vi "2.0.0_BEMF_Calibration.vi"(6 ".bat":T1={"getVersion"="Getting Software Version.bat", "Start Test mode"="Start Test Mode.bat", "Start camera test mode"="Start camera test mode.bat", "get one RAW Image"="Get one image.bat", "Stop camera test mode"="Stop camera test mode.bat", "Stop Test Mode"="Stop Test Mode.bat", "Get image reflection"="Get image reflection.bat", "Get image uniformity andFlash LED brightness"="Get image uniformity andFlash LED brightness.bat", "Disable flash LED"="Disable flash LED.bat", "Enable flash LED"="Enable flash LED.bat", "Software Reset"="Software Reset.bat", "Tune Flash LED brightness"="Tune Flash LED brightness.bat", "Start Camera calibration"="Start Camera calibration.bat", "Verify OBC Setting"="Verify OBC Setting.bat"}, 7 "Data in":T3, 8 "error in (no error)":errorcluster, 9 "AllControls In":T2, 11 "Message Queue out":T4) -> (0 "error out":errorcluster, 1 "Flow":string, 3 "Message Queue Out":T4, 5 "Data out":T3)   [LabVIEW 2017]
uses:
  Depends/AMC/subVIs/TypeDefs/amc_Message Queue.ctl
  Depends/AMC/subVIs/TypeDefs/amc_Message.ctl
  Depends/Tools/Keyed Array/Tools_KeyedArray KeyedArray.ctl
  Ctrls/CSV_Data.ctl
  Ctrls/AllControls.ctl
  Ctrls/NFC.bat
panel:
  out "GetImage?":bool
  out "retry_flag":bool
  in  "Num":i32
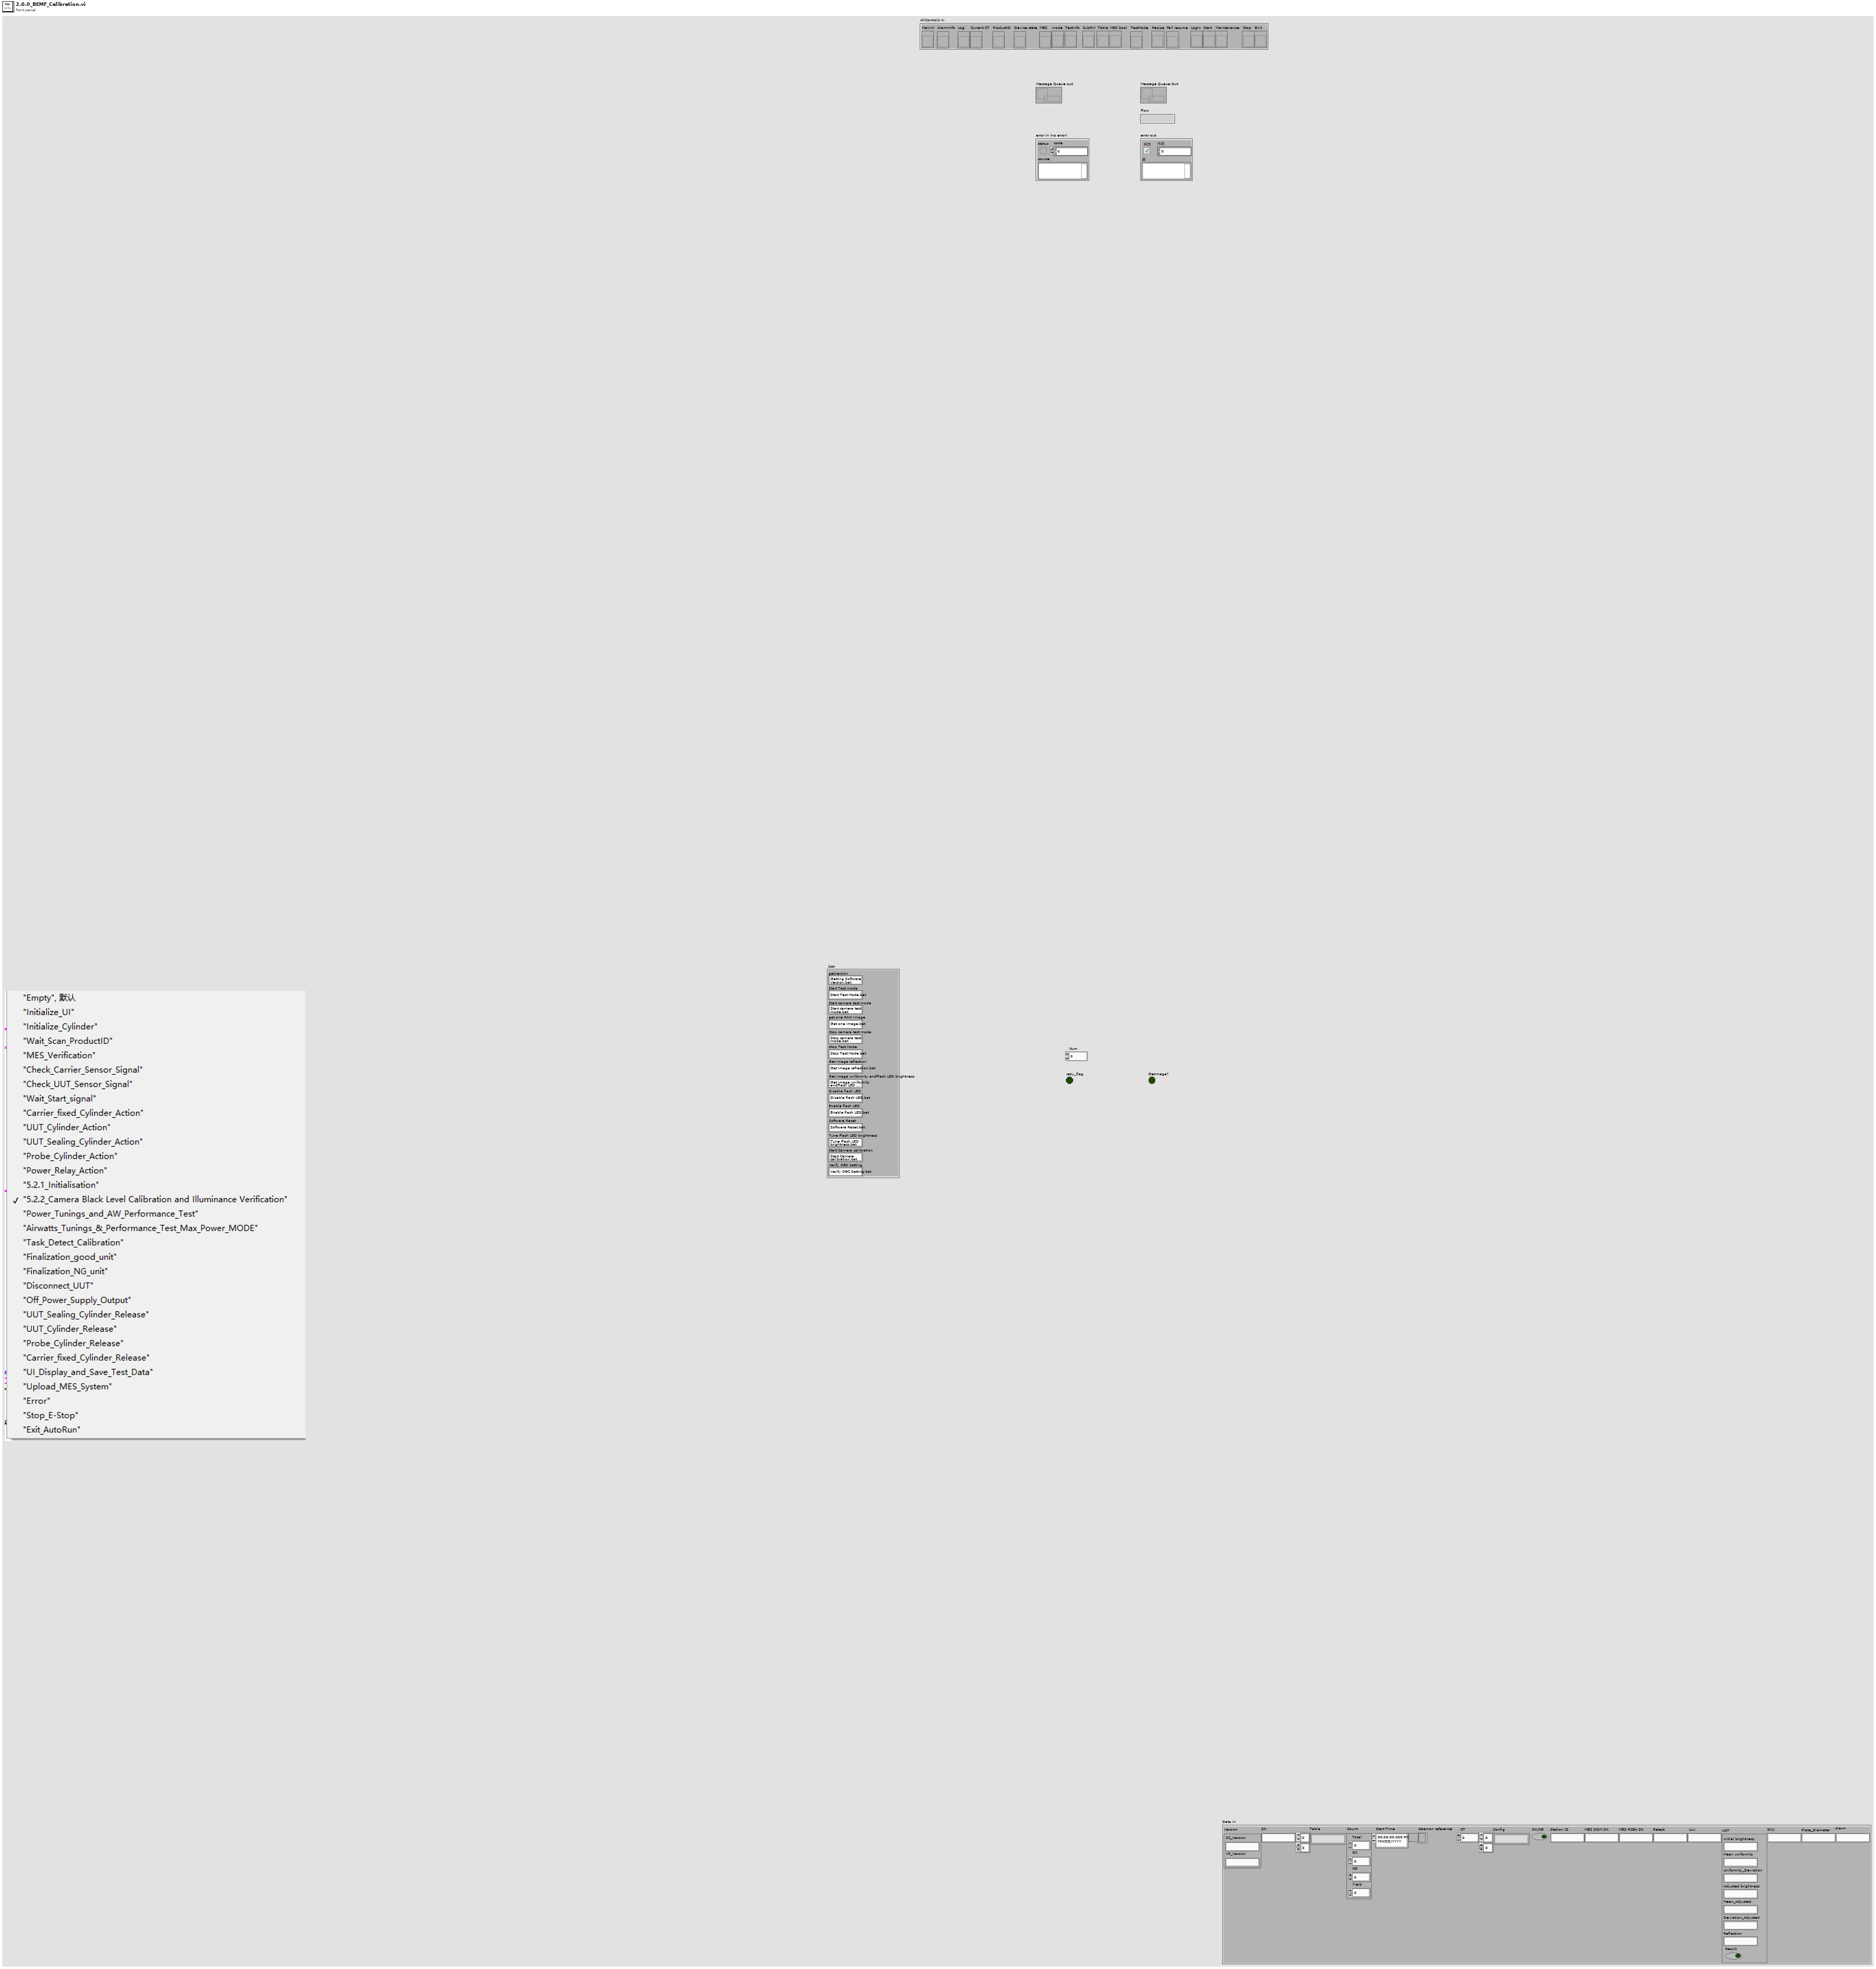
[diagram p1: front panel]
types:
  T1 = typedef "NFC.bat" = cluster{"getVersion":string, "Start Test mode":string, "Start camera test mode":string, "get one RAW Image":string, "Stop camera test mode":string, "Stop Test Mode":string, "Get image reflection":string, "Get image uniformity andFlash LED brightness":string, "Disable flash LED":string, "Enable flash LED":string, "Software Reset":string, "Tune Flash LED brightness":string, "Start Camera calibration":string, "Verify OBC Setting":string}
  T2 = typedef "AllControls.ctl" = cluster{"MainVI":refnum<vi>, "AlarmInfo":refnum<vi>, "Log":refnum<vi>, "Current CT":refnum<vi>, "ProductID":refnum<vi>, "Device state":refnum<vi>, "MES":refnum<vi>, "mode":refnum<vi>, "TestInfo":refnum<vi>, "SubPnl":refnum<vi>, "Table":refnum<vi>, "MES bool":refnum<vi>, "TestMode":refnum<vi>, "Recipe":refnum<vi>, "Fail resume":refnum<vi>, "LogIn":refnum<vi>, "Start":refnum<vi>, "Maintenance":refnum<vi>, "Stop":refnum<vi>, "Exit":refnum<vi>}
  T3 = typedef "CSV_Data.ctl" = cluster{"Version":cluster{"SC_Version":string, "VP_Version":string}, "SN":string, "Table":string[][], "Count":cluster{"Total":i32, "OK":i32, "NG":i32, "Yield":dbl}, "Start Time":timestamp, "daemon reference":refnum<k5>, "CT":dbl, "Config":string[][], "OK/NG":bool, "Station ID":string, "MES DDM SN":string, "MES PCBA SN":string, "Retest":string, "Lux":string, "VOT":cluster{"Initial brightness":string, "Mean uniformity":string, "Uniformity_Deviation":string, "Adjusted brightness":string, "Mean_Adjusted":string, "Deviation_Adjusted":string, "Reflection":string, "Result":bool}, "SKU":string, "Plate_Diameter":string, "Alarm":string}
  T4 = typedef "amc_Message Queue.ctl" = refnum<queue>
  T5 = typedef "HD Config.ctl" = cluster{" PC":cluster{"PC Address":u8[], "PC Port":i32}, "FCO":cluster{"COM":refnum<visa-resource-name>, "Baudrate":u32}, "DC Power ":cluster{"COM":refnum<visa-resource-name>, "Baudrate":u32}, "PW3336":cluster{"COM":refnum<visa-resource-name>, "Baudrate":u32}, "Lefoo":cluster{"COM":refnum<visa-resource-name>, "Baudrate":u32}, "Tempt&Hum":cluster{"COM":refnum<visa-resource-name>, "Baudrate":u32}, "DIPC":cluster{"COM":refnum<visa-resource-name>}, "Daemon":cluster{"IP Address":string, "Port":u16, "Retry":u16}, "NFC_Cmd":cluster{"COM":refnum<visa-resource-name>, "Baudrate":u32}, "Fail_resume_mode":bool, "GRR":bool, "NFC _Serial":cluster{"COM":refnum<visa-resource-name>, "Baudrate":u32}}
  T6 = typedef "TesterInfo.ctl" = cluster{"Station Name":string, "Station Code":string, "ES NO.":string, "Tester ID":string, "PassMark Revision":string, "Rig ID":string, "682_Tool_Repeat":string, "Project Name":string, "FFTesterPath":path, "Enable_User":bool, "Mode":enum16{"682"}, "Fail_resume_mode":bool}
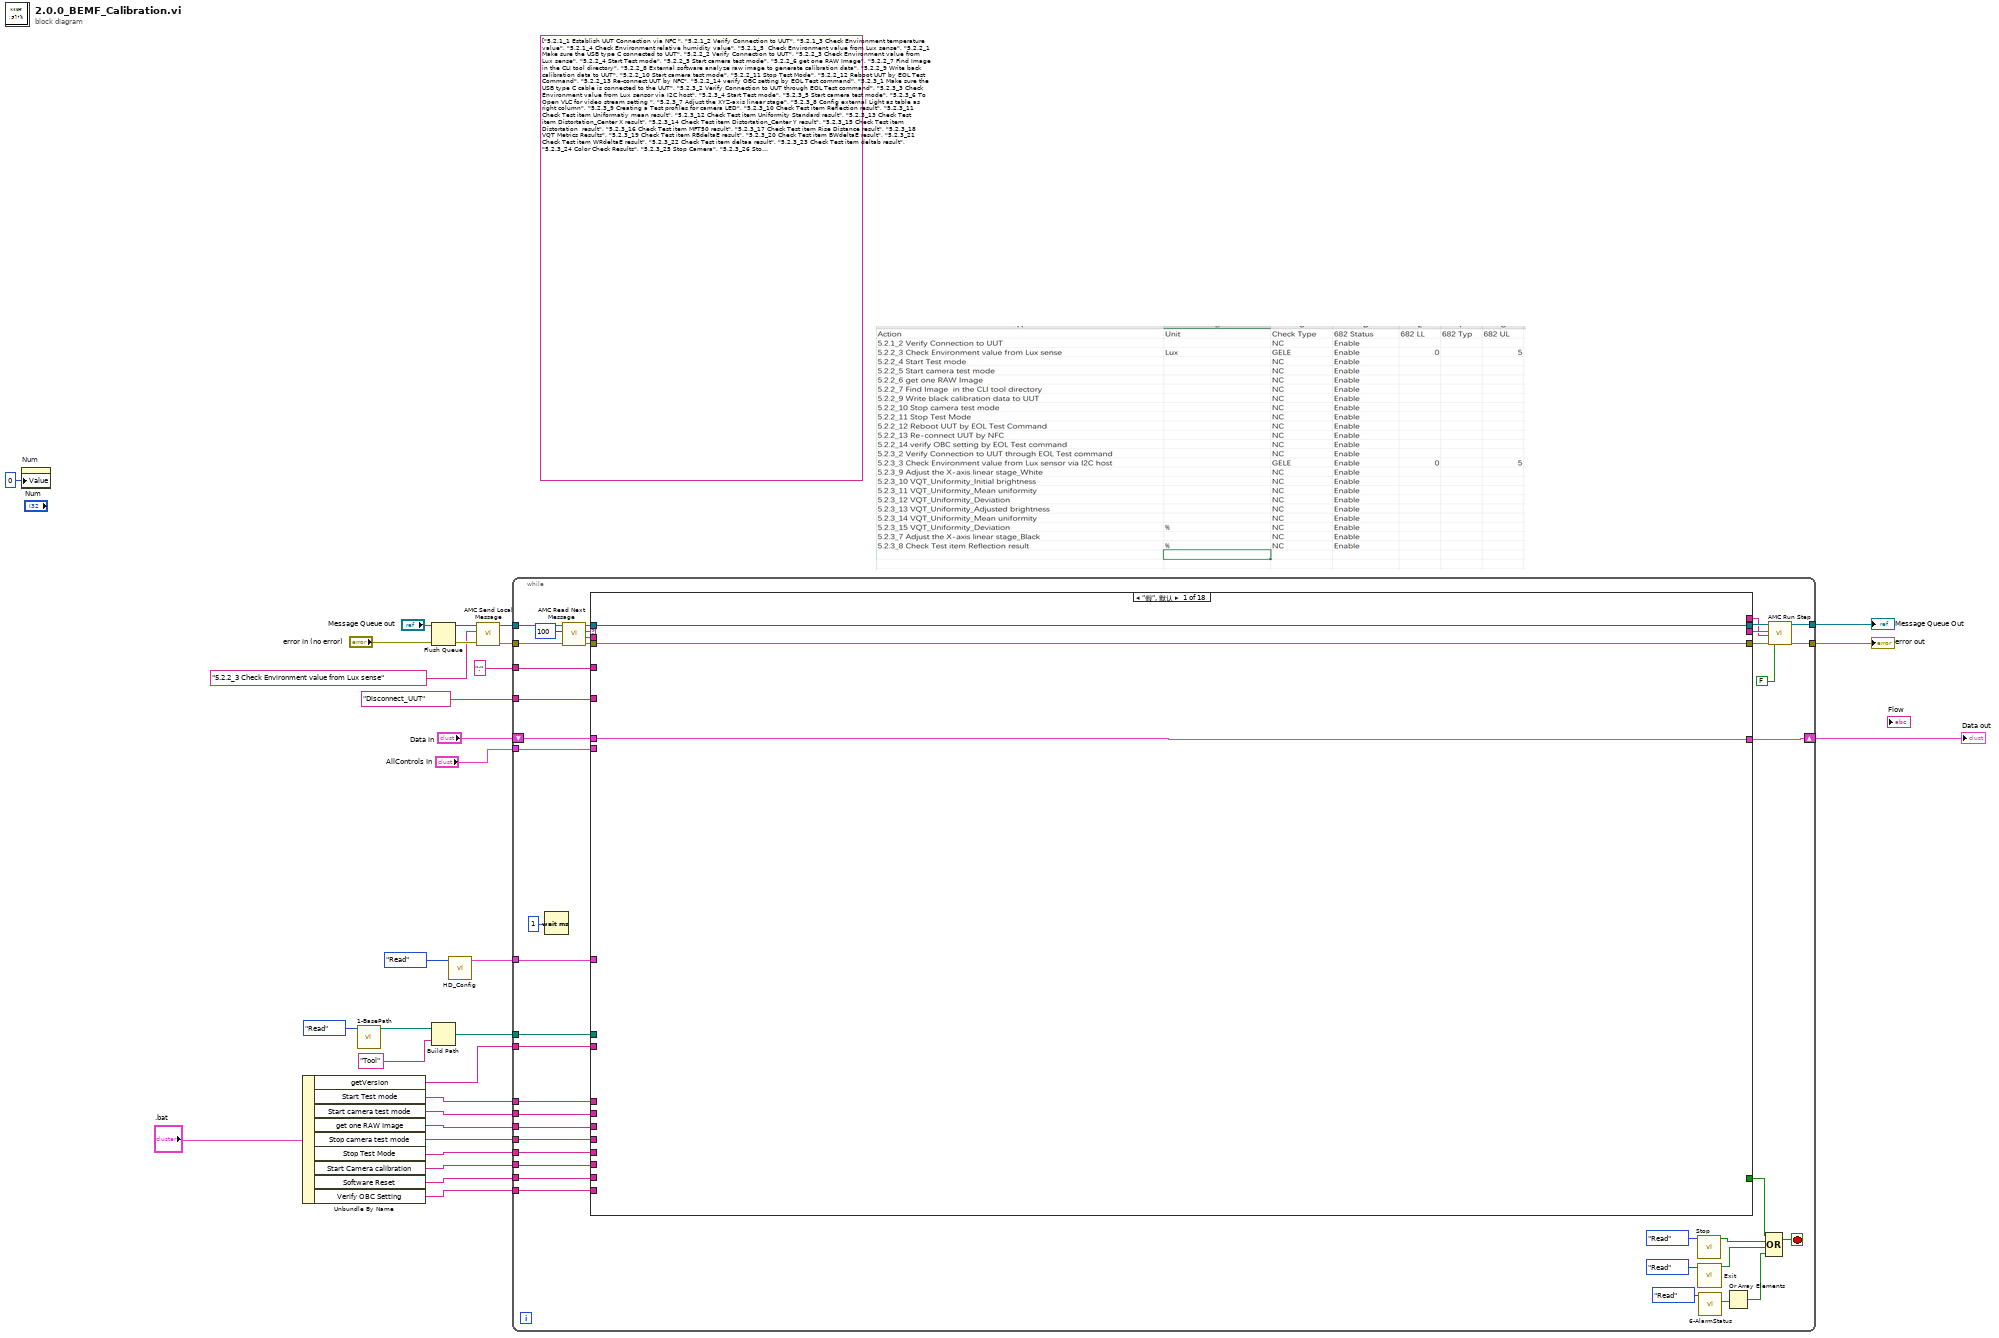
[diagram p0: block diagram]
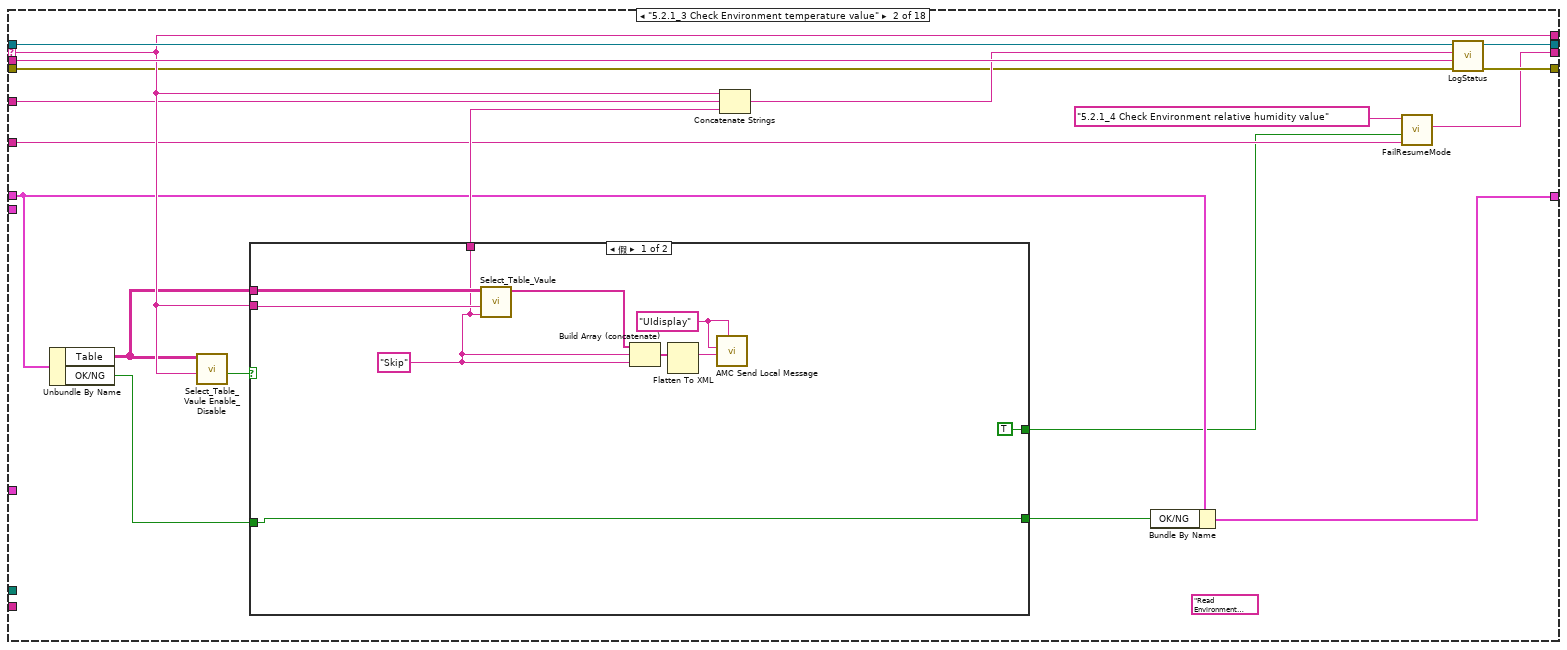
[diagram p2: hidden frame]
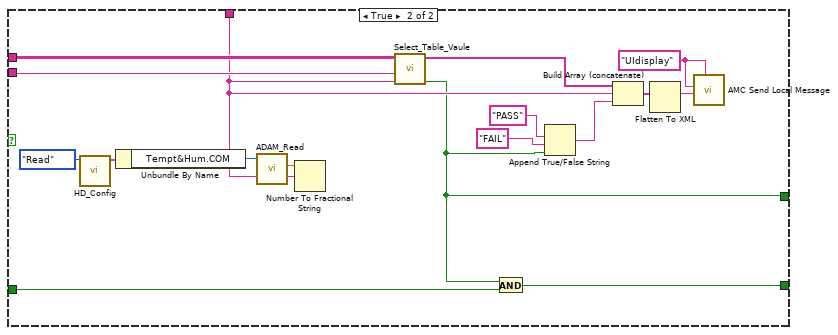
[diagram p3: hidden frame]
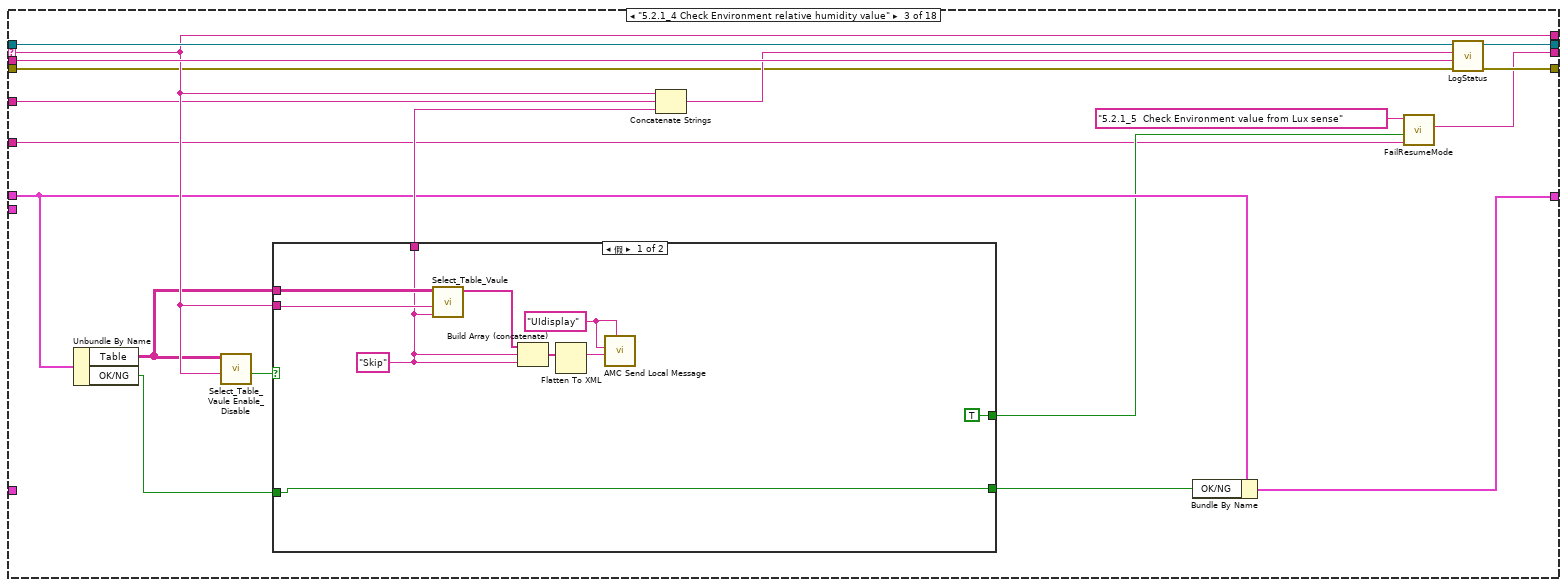
[diagram p4: hidden frame]
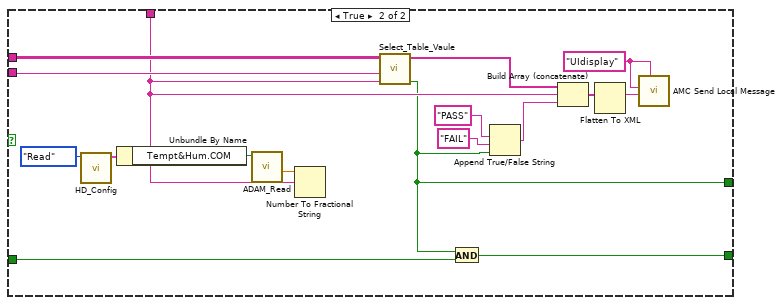
[diagram p5: hidden frame]
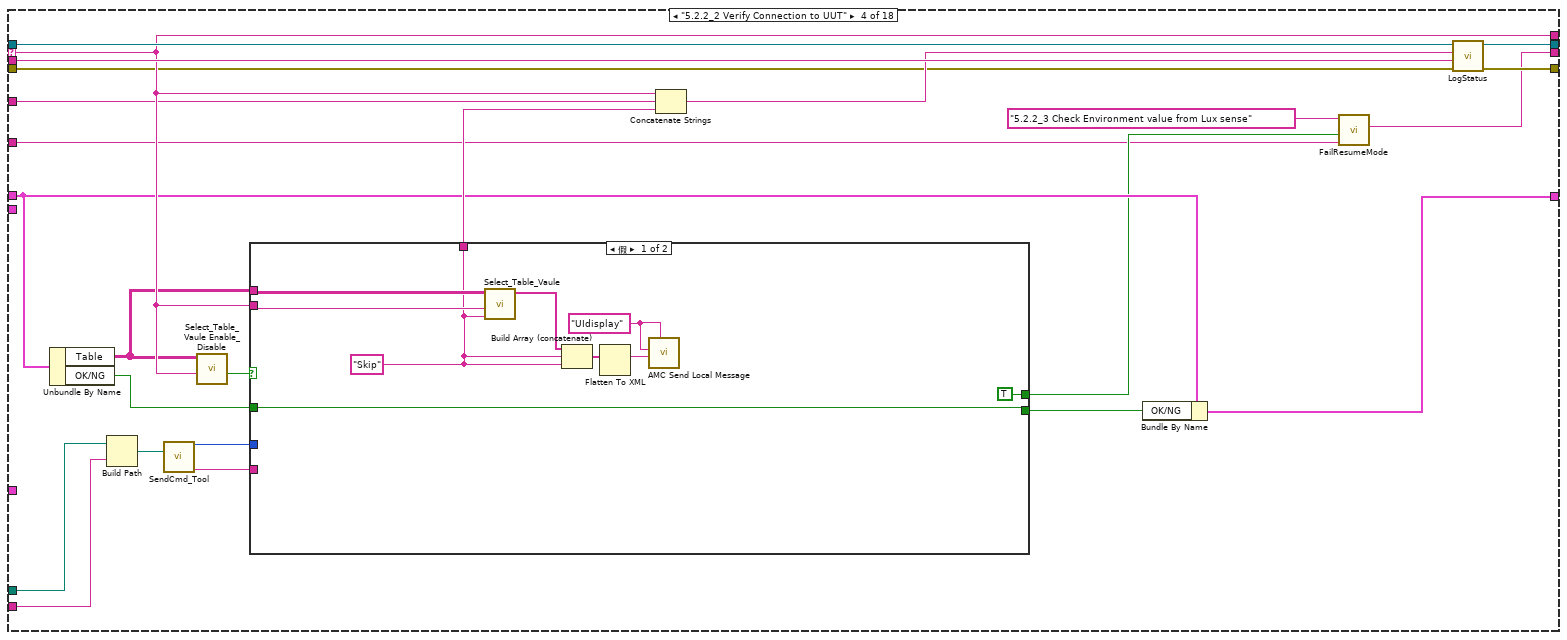
[diagram p6: hidden frame]
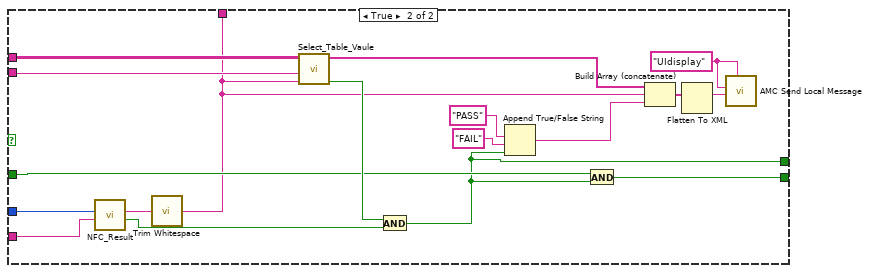
[diagram p7: hidden frame]
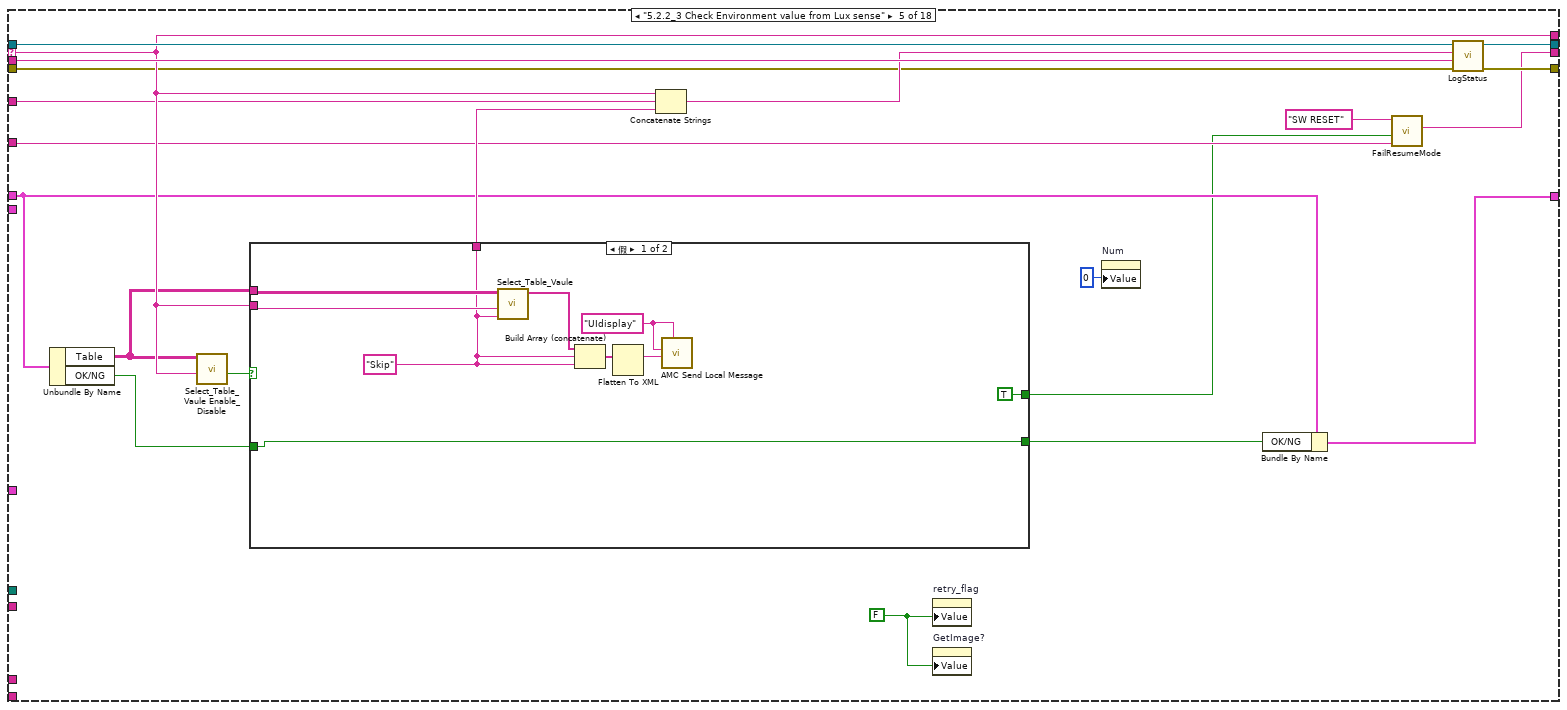
[diagram p8: hidden frame]
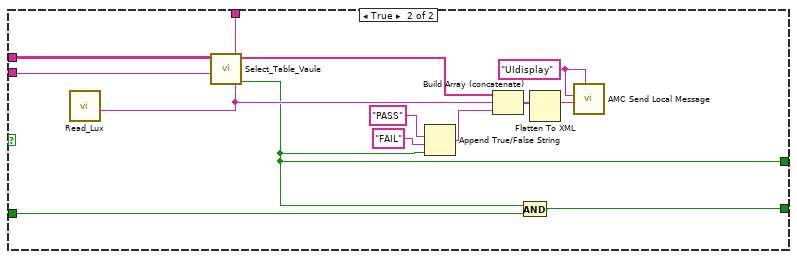
[diagram p9: hidden frame]
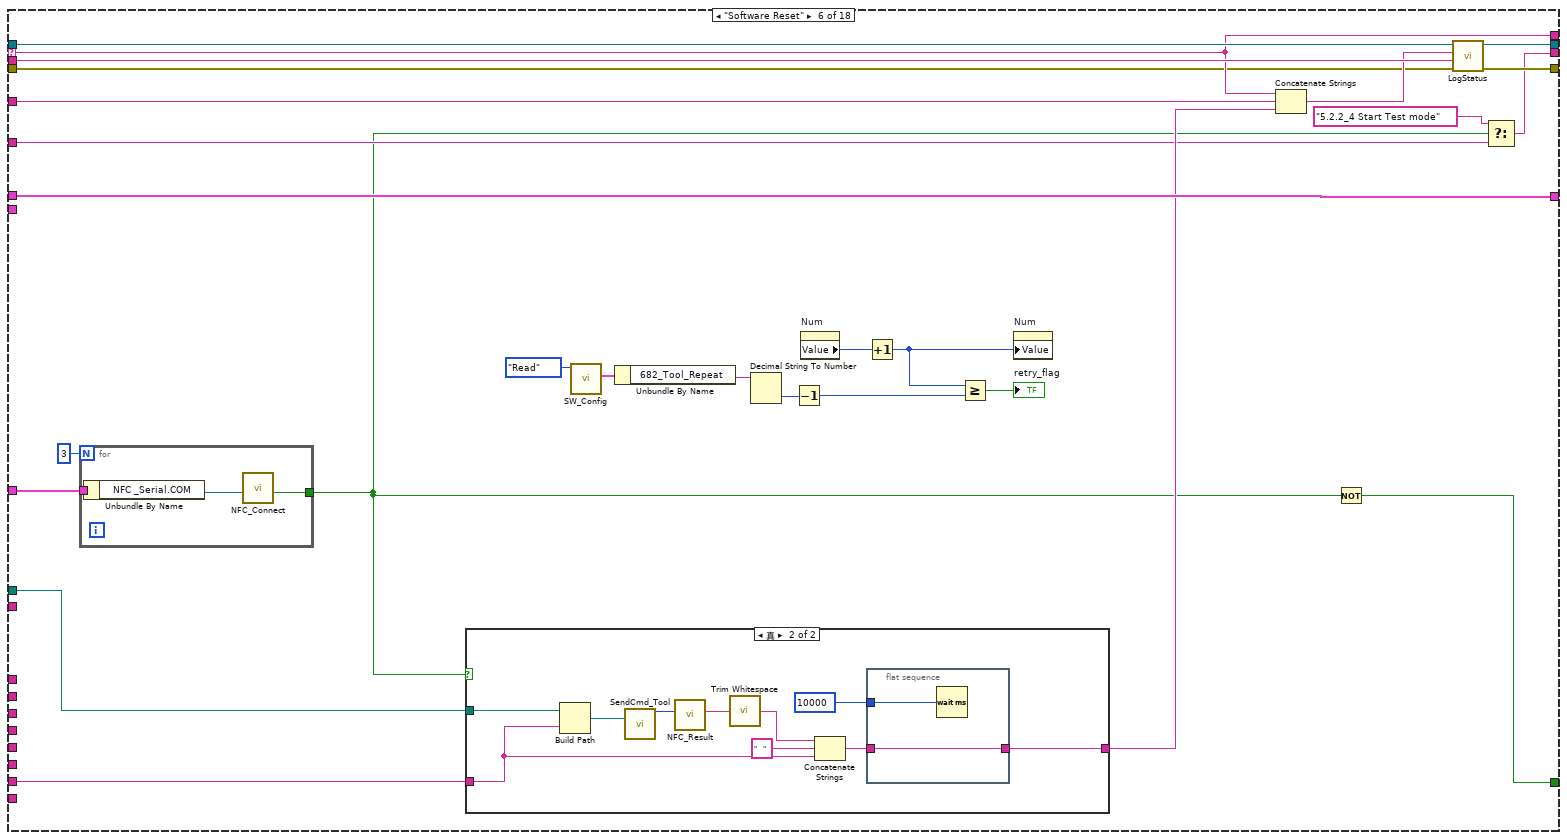
[diagram p10: hidden frame]
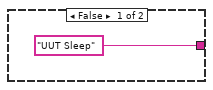
[diagram p11: hidden frame]
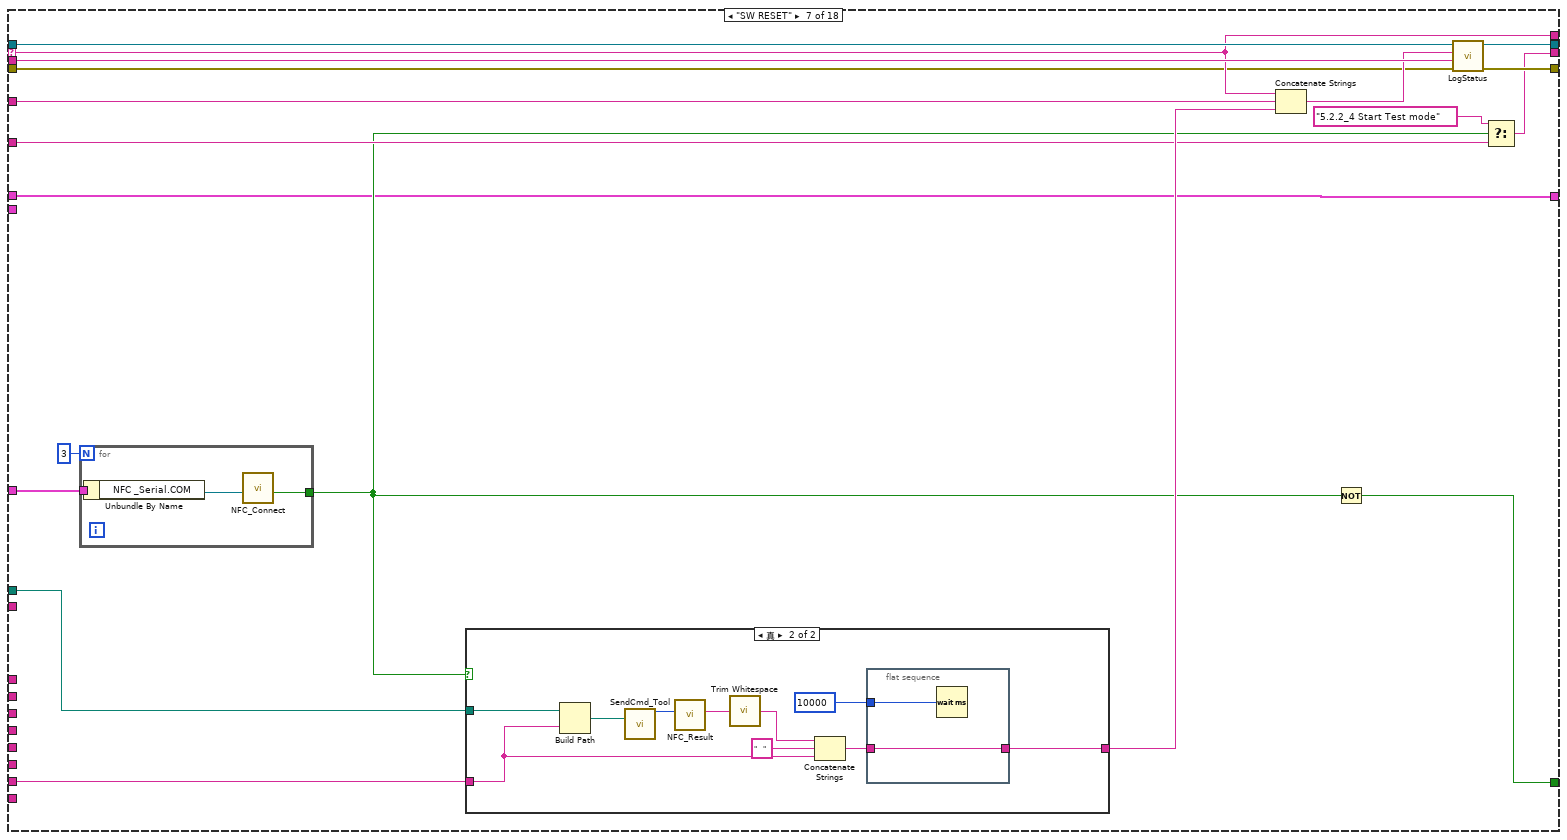
[diagram p12: hidden frame]
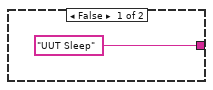
[diagram p13: hidden frame]
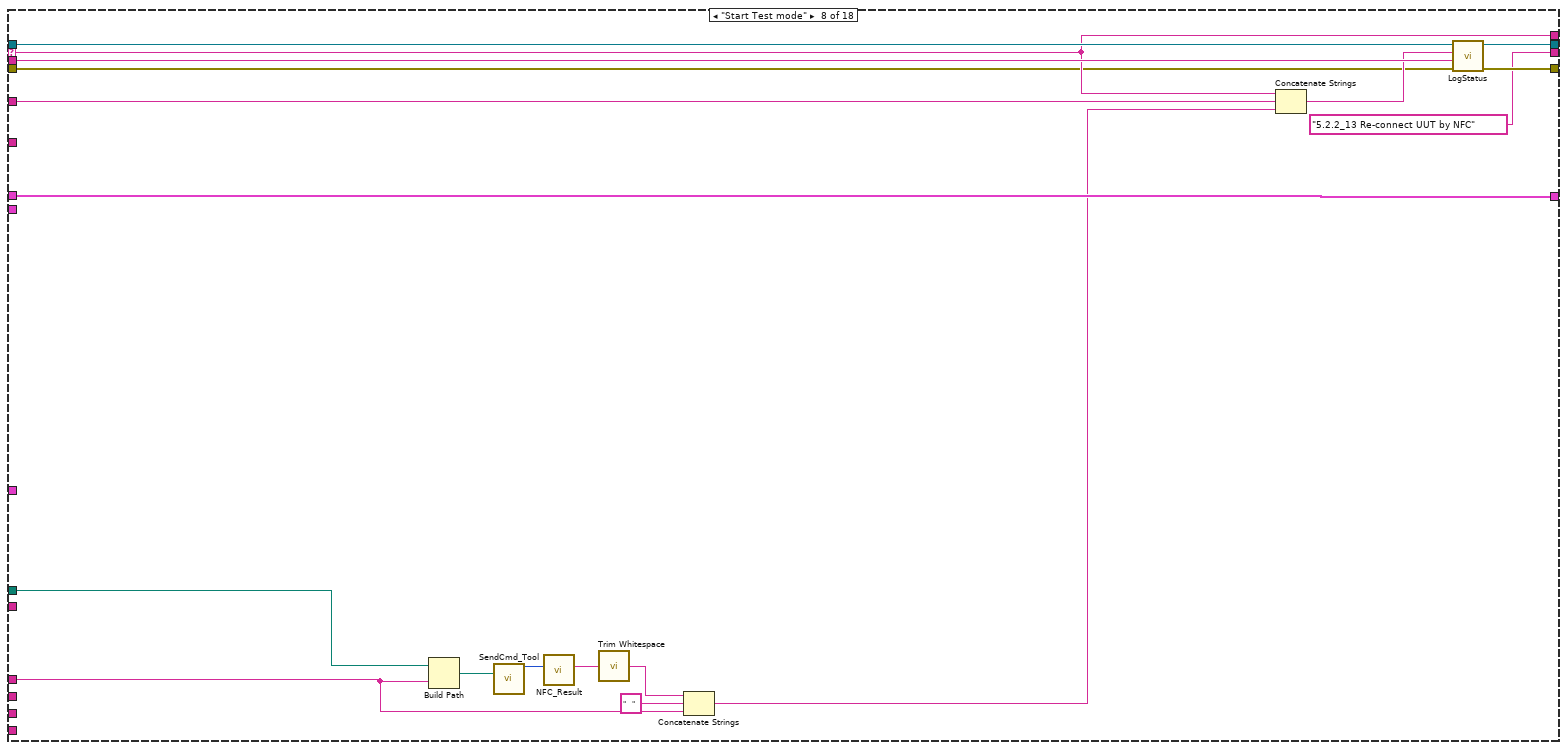
[diagram p14: hidden frame]
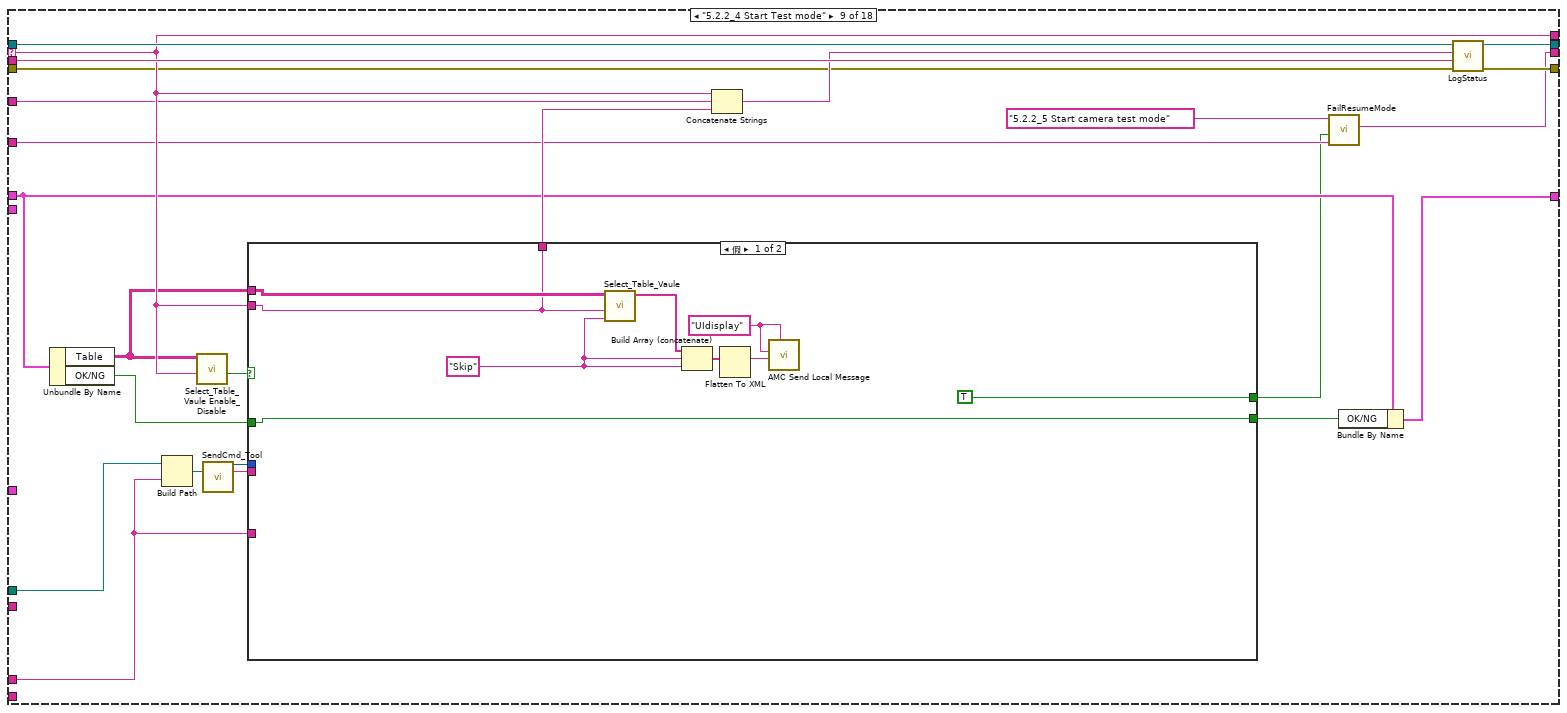
[diagram p15: hidden frame]
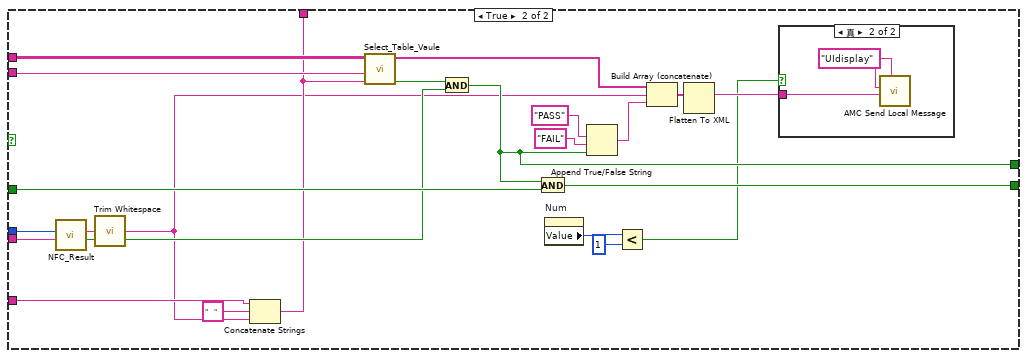
[diagram p16: hidden frame]
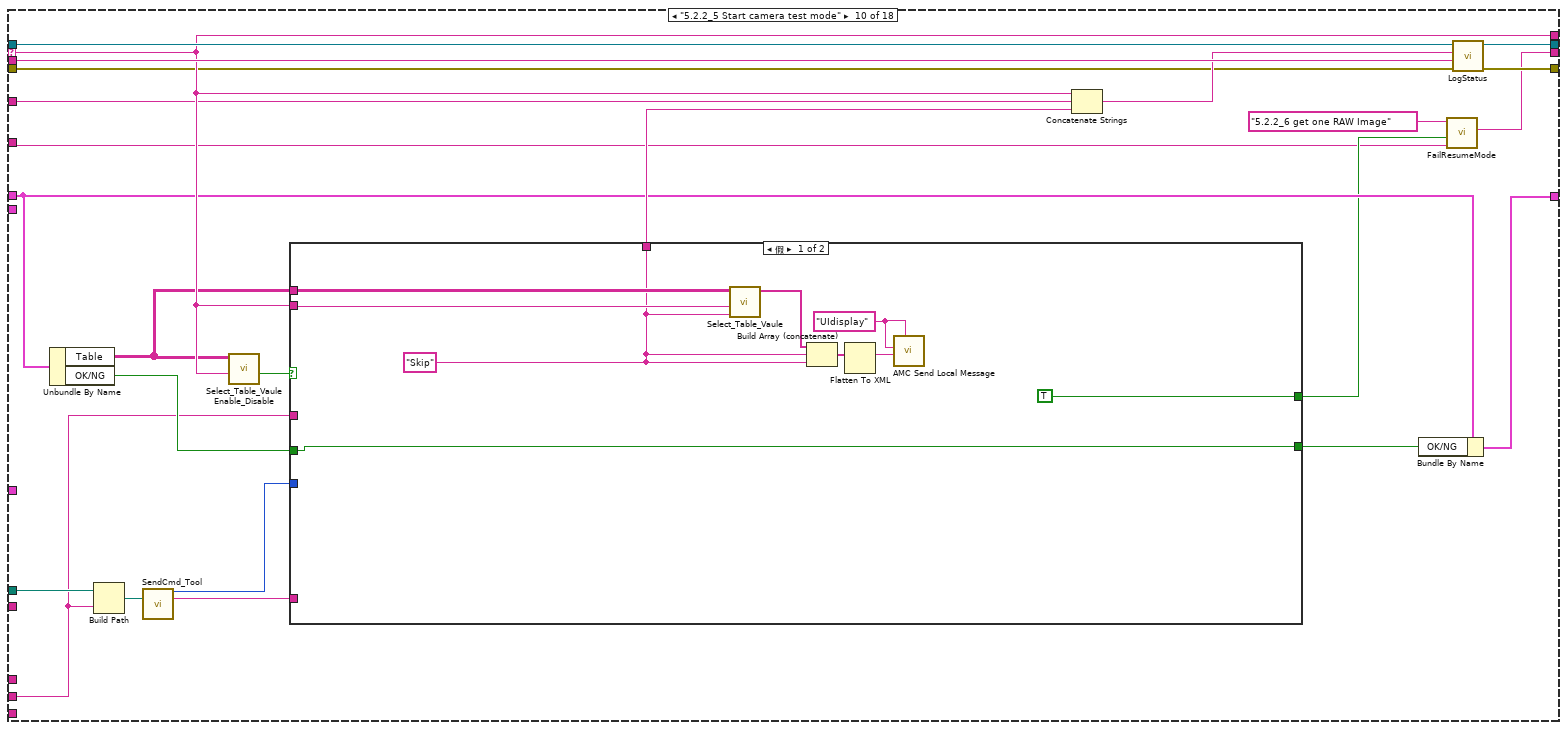
[diagram p18: hidden frame]
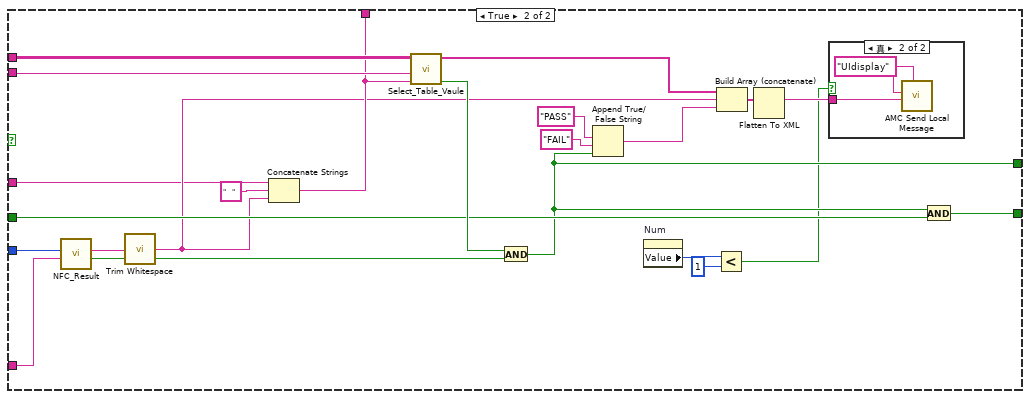
[diagram p19: hidden frame]
diagram:
  (unwired) string[] ["5.2.1_1 Establish UUT Connection via NFC ", "5.2.1_2 Verify Connection to UUT", "5.2.1_3 Check Environment temperature value", "5.2.1_4 Check Environment relative humidity value", "5.2.1_5  Check Environment value from Lux sense", "5.2.2_1 Make sure the USB type C connected to UUT", "5.2.2_2 Verify Connection to UUT", "5.2.2_3 Check Environment value from Lux sense", "5.2.2_4 Start Test mode", "5.2.2_5 Start camera test mode", "5.2.2_6 get one RAW Image", "5.2.2_7 Find Image  in the CLI tool directory", "5.2.2_8 External software analyze raw image to generate calibration data", "5.2.2_9 Write back calibration data to UUT", "5.2.2_10 Start camera test mode", "5.2.2_11 Stop Test Mode", "5.2.2_12 Reboot UUT by EOL Test Command", "5.2.2_13 Re-connect UUT by NFC", "5.2.2_14 verify OBC setting by EOL Test command", "5.2.3_1 Make sure the USB type C cable is connected to the UUT", "5.2.3_2 Verify Connection to UUT through EOL Test command", "5.2.3_3 Check Environment value from Lux sensor via I2C host", "5.2.3_4 Start Test mode", "5.2.3_5 Start camera test mode", "5.2.3_6 To Open VLC for video stream setting ", "5.2.3_7 Adjust the XYZ-axis linear stage", "5.2.3_8 Config external Light as table as right column", "5.2.3_9 Creating a Test profiles for camera LED", "5.2.3_10 Check Test item Reflection result", "5.2.3_11 Check Test item Uniformatiy mean result", "5.2.3_12 Check Test item Uniformity Standard result", "5.2.3_13 Check Test item Distortation_Center X result", "5.2.3_14 Check Test item Distortation_Center Y result", "5.2.3_15 Check Test item Distortation  result", "5.2.3_16 Check Test item MFT50 result", "5.2.3_17 Check Test item Rise Distance result", "5.2.3_18 VQT Metrics Results", "5.2.3_19 Check Test item RBdeltaE result", "5.2.3_20 Check Test item BWdeltaE result", "5.2.3_21 Check Test item WRdeltaE result", "5.2.3_22 Check Test item deltaa result", "5.2.3_23 Check Test item deltab result", "5.2.3_24 Color Check Results", "5.2.3_25 Stop Camera", "5.2.3_26 Stop Test mode", "5.2.3_27 Shutdown UUT"] ("subarray")
  n1 = property on="Num" class="DigNum (严格)"("Value"=0 ("Num")) -> ()  [unwired: 2 in, 2 out]
  n2 = Unbundle By Name(".bat") -> ("getVersion"=w14:string, "Start Test mode"=w13:string, "Start camera test mode"=w12:string, "get one RAW Image"=w11:string, "Stop camera test mode"=w10:string, "Stop Test Mode"=w9:string, "Start Camera calibration"=w6:string, "Software Reset"=w4:string, "Verify OBC Setting"=w3:string)
  n3 = call "1-BasePath.vi"("Step"=enum16{"Initial", "Write", "Read"}."Read") -> ("Path Out"=w16:path)  [unwired: 9 in, 1 out]
  n4 = Flush Queue(queue="Message Queue out") -> (queue out=w24:T4)  [unwired: 1 in, 2 out]
  n5 = Build Path(base path=w16, name or relative path="Tool") -> (appended path=w15:path)
  n6 = call "HD_Config.vi"("Step"=enum16{"Initial", "Write", "Read"}."Read") -> ("HD Config out"=w25:T5)  [unwired: 9 in, 1 out]
  n7 = call "AMC Send Local Message.vi"("error in (no error)"="error in (no error)", "Message Name"="5.2.2_3 Check Environment value from Lux sense", "Message Queue in"=w24) -> ("error out"=w28:errorcluster, "Message Queue out"=w29:T4)  [unwired: 7 in]
  n8 = while {
    tunnel: w29 -> [w70]
    tunnel: [w66] -> w23
    tunnel: w28 -> [w64]
    tunnel: [w61] -> w22
    tunnel: w25 -> [w58]
    shift-right: [w47] -> w20
    shift-left: "Data in" -> [w48]
    tunnel: "AllControls In" -> [w46]
    tunnel: w15 -> [w42]
    tunnel: w14 -> [w41]
    tunnel: w13 -> [w40]
    tunnel: w12 -> [w39]
    tunnel: w11 -> [w38]
    tunnel: w10 -> [w37]
    tunnel: w9 -> [w36]
    tunnel: ":" -> [w35]
    tunnel: "Disconnect_UUT" -> [w34]
    tunnel: w6 -> [w33]
    tunnel: w4 -> [w32]
    tunnel: w3 -> [w31]
    stop <- w49 stop-if-true
    n9 = Wait (ms)(milliseconds to wait=u32 1 ("等待时间（毫秒）")) -> ()  [unwired: 1 out]
    n10 = call "AMC Read Next Message.vi"("error in (no error)"=w64, "timeout (1ms)"=100, "Message Queue in"=w70) -> ("error out"=w63:errorcluster, "Message Value"=w56:string, "Message Name"=w68:string, "Message Queue out"=w69:T4)  [unwired: 1 in, 4 out]
    n11 = case shown="\"假\", 默认" w68 {
      selector: w68 -> [_ w85 w129 w178 w225 w275 w309 w342 w363 w420 w483 w537 w584 w638 w688 w738 w794 w846]
      tunnel: w69 -> [w73 w91 w135 w184 w231 w279 w313 w346 w369 w426 w489 w543 w590 w644 w694 w742 w799 w851]
      tunnel: [w73 w91 w135 w184 w231 w279 w313 w346 w369 w426 w489 w543 w590 w644 w694 w742 w799 w851] -> w67
      tunnel: w63 -> [w72 w79 w123 w167 w219 w274 w308 w341 w353 w410 w476 w535 w582 w627 w677 w736 w792 w843]
      tunnel: [w72 w90 w134 w183 w230 w278 w312 w345 w368 w425 w488 w542 w589 w643 w693 w741 w798 w850] -> w62
      tunnel: [_ _ _ _ _ w260 w299 _ _ _ _ _ _ _ _ _ _ TRUE] -> w50
      tunnel: w56 -> [_ w89 w133 w182 w229 w277 w311 w344 w367 w424 w487 w541 w588 w642 w692 w740 w797 w849]
      tunnel: [_ w85 w129 w178 w225 w275 w309 w342 w363 w420 w483 w537 w584 w638 w688 w738 w794 w846] -> w55
      tunnel: w58 -> [_ _ _ _ _ w264 w296 _ _ _ _ _ _ _ _ w733 w788 _]
      tunnel: [_ w75 w118 w162 w216 w262 w301 "5.2.2_13 Re-connect UUT by NFC" w349 w405 w473 w526 w568 w622 w672 w723 w781 w840] -> w57
      tunnel: w48 -> [w71 w83 w126 w170 w223 w271 w297 w338 w356 w415 w478 w532 w575 w630 w680 w728 w787 w836]
      tunnel: [w71 w80 w124 w169 w220 w271 w297 w338 w355 w414 w477 w530 w574 w629 w679 w727 w785 w834] -> w47
      tunnel: w46 -> [_ _ _ _ _ _ _ _ _ _ _ _ _ _ _ _ _ _]
      tunnel: w42 -> [_ _ _ w175 _ w272 w306 w339 w360 w417 w472 _ w578 w635 w685 w731 _ w838]
      tunnel: w41 -> [_ _ _ w174 _ _ _ _ _ _ _ _ _ _ _ _ _ _]
      tunnel: w40 -> [_ _ _ _ _ _ _ w336 w348 _ _ _ _ _ _ _ _ _]
      tunnel: w39 -> [_ _ _ _ _ _ _ _ _ w404 _ _ _ _ _ _ _ _]
      tunnel: w38 -> [_ _ _ _ _ _ _ _ _ _ w461 _ _ _ _ _ _ _]
      tunnel: w37 -> [_ _ _ _ _ _ _ _ _ _ _ _ _ w634 _ _ _ _]
      tunnel: w36 -> [_ _ _ _ _ _ _ _ _ _ _ _ _ _ w684 _ _ _]
      tunnel: w35 -> [_ w78 w122 w166 w218 w273 w307 w340 w352 w409 w475 w534 w581 w626 w676 w735 w791 w842]
      tunnel: w34 -> [_ w76 w120 w163 w217 w263 w302 _ w350 w406 w474 w533 w571 w624 w673 w734 w790 w839]
      tunnel: w33 -> [_ _ _ _ _ _ _ _ _ _ _ _ w570 _ _ _ _ _]
      tunnel: w32 -> [_ _ _ _ _ w270 w305 _ _ _ _ _ _ _ _ w730 _ _]
      tunnel: w31 -> [_ _ _ _ _ _ _ _ _ _ _ _ _ _ _ _ _ w837]
      frame "假", Default {
      }
      frame "5.2.1_3 Check Environment temperature value" {
        (unwired) "Read Environment Illuminance Value Success"
        n12 = Unbundle By Name(w83) -> ("Table"=w84:string[][], "OK/NG"=w82:bool)
        n13 = call "Select_Table_Vaule Enable_Disable.vi"("Action"=w85, "Table"=w84) -> ("Enable"=w86:bool)  [unwired: 8 in, 1 out]
        n14 = case shown="假" w86 {
          tunnel: [w93 w105] -> w87
          tunnel: w85 -> [w94 w112]
          tunnel: w84 -> [w95 w111]
          tunnel: w82 -> [w92 w103]
          tunnel: [w92 w102] -> w81
          tunnel: [TRUE ("Result") w101] -> w74
          frame False {
            w99 = "UIdisplay" ("Process (\"\" - local)")
            w93 = "Skip" ("Action")
            n15 = call "Select_Table_Vaule.vi"("Vaule"=w93, "Action"=w94, "Table"=w95) -> ("vaule"=w96:string[])  [unwired: 7 in, 1 out]
            n16 = Build Array (concatenate)(w96, w93, w93) -> (w98:string[])
            n17 = Flatten To XML(anything=w98) -> (xml string=w97:string)
            n18 = call "AMC Send Local Message.vi"("Process (\"\" - local)"=w99, "Message Value"=w97, "Message Name"=w99) -> ()  [unwired: 7 in, 2 out]
          }
          frame True {
            w117 = "UIdisplay" ("Process (\"\" - local)")
            n19 = call "HD_Config.vi"("Step"=enum16{"Initial", "Write", "Read"}."Read") -> ("HD Config out"=w108:T5)  [unwired: 9 in, 1 out]
            n20 = Unbundle By Name(w108) -> ("Tempt&Hum.COM"=w106:refnum<visa-resource-name>)
            n21 = call "ADAM_Read.vi"("VISA resource name"=w106) -> ("temperature"=w104:dbl)  [unwired: 7 in, 3 out]
            n22 = Number To Fractional String(number=w104) -> (F-format string=w105:string)  [unwired: 3 in]
            n23 = call "Select_Table_Vaule.vi"("Vaule"=w105, "Action"=w112, "Table"=w111) -> ("Result"=w101:bool, "vaule"=w110:string[])  [unwired: 7 in]
            n24 = And(x=w101, y=w103) -> (x .and. y?=w102:bool)
            n25 = Append True/False String(1:w101, 2:"FAIL" ("真字符串"), 3:"PASS" ("真字符串")) -> (0:w109:string)  [unwired: 1 in]
            n26 = Build Array (concatenate)(w110, w105, w109) -> (w116:string[])
            n27 = Flatten To XML(anything=w116) -> (xml string=w115:string)
            n28 = call "AMC Send Local Message.vi"("Process (\"\" - local)"=w117, "Message Value"=w115, "Message Name"=w117) -> ()  [unwired: 7 in, 2 out]
          }
        }
        n29 = Concatenate Strings(w85, w78, w87) -> (w88:string)
        n30 = Bundle By Name(cluster=w83, "OK/NG"=w81) -> (w80:T3)
        n31 = call "FailResumeMode.vi"("NextMessage"="5.2.1_4 Check Environment relative humidity value", "OK/NG"=w74, "EndMessage"=w76) -> ("OutMessage"=w75:string)  [unwired: 6 in]
        n32 = call "LogStatus.vi"("error in (no error)"=w79, "last message"=w89, "message"=w88) -> ("error  out"=w90:errorcluster)  [unwired: 8 in]
      }
      frame "5.2.1_4 Check Environment relative humidity value" {
        n33 = Unbundle By Name(w126) -> ("Table"=w128:string[][], "OK/NG"=w127:bool)
        n34 = call "Select_Table_Vaule Enable_Disable.vi"("Action"=w129, "Table"=w128) -> ("Enable"=w130:bool)  [unwired: 8 in, 1 out]
        n35 = case shown="假" w130 {
          tunnel: [w137 w149] -> w131
          tunnel: w129 -> [w138 w156]
          tunnel: w128 -> [w139 w155]
          tunnel: w127 -> [w136 w147]
          tunnel: [w136 w146] -> w125
          tunnel: [TRUE ("Result") w145] -> w121
          frame False {
            w143 = "UIdisplay" ("Process (\"\" - local)")
            w137 = "Skip" ("Action")
            n36 = call "Select_Table_Vaule.vi"("Vaule"=w137, "Action"=w138, "Table"=w139) -> ("vaule"=w140:string[])  [unwired: 7 in, 1 out]
            n37 = Build Array (concatenate)(w140, w137, w137) -> (w142:string[])
            n38 = Flatten To XML(anything=w142) -> (xml string=w141:string)
            n39 = call "AMC Send Local Message.vi"("Process (\"\" - local)"=w143, "Message Value"=w141, "Message Name"=w143) -> ()  [unwired: 7 in, 2 out]
          }
          frame True {
            w161 = "UIdisplay" ("Process (\"\" - local)")
            n40 = call "HD_Config.vi"("Step"=enum16{"Initial", "Write", "Read"}."Read") -> ("HD Config out"=w152:T5)  [unwired: 9 in, 1 out]
            n41 = Unbundle By Name(w152) -> ("Tempt&Hum.COM"=w150:refnum<visa-resource-name>)
            n42 = call "ADAM_Read.vi"("VISA resource name"=w150) -> ("humidity"=w148:dbl)  [unwired: 7 in, 3 out]
            n43 = Number To Fractional String(number=w148) -> (F-format string=w149:string)  [unwired: 3 in]
            n44 = call "Select_Table_Vaule.vi"("Vaule"=w149, "Action"=w156, "Table"=w155) -> ("Result"=w145:bool, "vaule"=w154:string[])  [unwired: 7 in]
            n45 = And(x=w145, y=w147) -> (x .and. y?=w146:bool)
            n46 = Append True/False String(1:w145, 2:"FAIL" ("真字符串"), 3:"PASS" ("真字符串")) -> (0:w153:string)  [unwired: 1 in]
            n47 = Build Array (concatenate)(w154, w149, w153) -> (w160:string[])
            n48 = Flatten To XML(anything=w160) -> (xml string=w159:string)
            n49 = call "AMC Send Local Message.vi"("Process (\"\" - local)"=w161, "Message Value"=w159, "Message Name"=w161) -> ()  [unwired: 7 in, 2 out]
          }
        }
        n50 = Concatenate Strings(w129, w122, w131) -> (w132:string)
        n51 = Bundle By Name(cluster=w126, "OK/NG"=w125) -> (w124:T3)
        n52 = call "FailResumeMode.vi"("NextMessage"="5.2.1_5  Check Environment value from Lux sense", "OK/NG"=w121, "EndMessage"=w120) -> ("OutMessage"=w118:string)  [unwired: 6 in]
        n53 = call "LogStatus.vi"("error in (no error)"=w123, "last message"=w133, "message"=w132) -> ("error  out"=w134:errorcluster)  [unwired: 8 in]
      }
      frame "5.2.2_2 Verify Connection to UUT" {
        n54 = Unbundle By Name(w170) -> ("Table"=w177:string[][], "OK/NG"=w171:bool)
        n55 = Build Path(base path=w175, name or relative path=w174) -> (appended path=w176:path)
        n56 = call "SendCmd_Tool.vi"("path_bat"=w176) -> ("return code"=w173:i32, "version info"=w172:string)  [unwired: 7 in, 6 out]
        n57 = call "Select_Table_Vaule Enable_Disable.vi"("Action"=w178, "Table"=w177) -> ("Enable"=w179:bool)  [unwired: 8 in, 1 out]
        n58 = case shown="假" w179 {
          tunnel: [w186 w199] -> w180
          tunnel: w178 -> [w187 w206]
          tunnel: w177 -> [w188 w205]
          tunnel: w173 -> [_ w198]
          tunnel: w172 -> [_ w197]
          tunnel: w171 -> [w185 w201]
          tunnel: [w185 w200] -> w168
          tunnel: [TRUE w194] -> w164
          frame False {
            w192 = "UIdisplay" ("Process (\"\" - local)")
            w186 = "Skip" ("Action")
            n59 = call "Select_Table_Vaule.vi"("Vaule"=w186, "Action"=w187, "Table"=w188) -> ("vaule"=w189:string[])  [unwired: 7 in, 1 out]
            n60 = Build Array (concatenate)(w189, w186, w186) -> (w191:string[])
            n61 = Flatten To XML(anything=w191) -> (xml string=w190:string)
            n62 = call "AMC Send Local Message.vi"("Process (\"\" - local)"=w192, "Message Value"=w190, "Message Name"=w192) -> ()  [unwired: 7 in, 2 out]
          }
          frame True {
            w211 = "UIdisplay" ("Process (\"\" - local)")
            n63 = call "NFC_Result.vi"("input"=w197, "return code"=w198) -> ("Command Sucess"=w196:bool, "return_result"=w195:string)  [unwired: 8 in]
            n64 = call <vilib>:"Trim Whitespace.vi"("string"=w195) -> ("trimmed string"=w199:string)  [unwired: 1 in]
            n65 = call "Select_Table_Vaule.vi"("Vaule"=w199, "Action"=w206, "Table"=w205) -> ("Result"=w202:bool, "vaule"=w204:string[])  [unwired: 7 in]
            n66 = And(x=w202, y=w196) -> (x .and. y?=w194:bool)
            n67 = Append True/False String(1:w194, 2:"FAIL" ("真字符串"), 3:"PASS" ("真字符串")) -> (0:w203:string)  [unwired: 1 in]
            n68 = And(x=w201, y=w194) -> (x .and. y?=w200:bool)
            n69 = Build Array (concatenate)(w204, w199, w203) -> (w210:string[])
            n70 = Flatten To XML(anything=w210) -> (xml string=w209:string)
            n71 = call "AMC Send Local Message.vi"("Process (\"\" - local)"=w211, "Message Value"=w209, "Message Name"=w211) -> ()  [unwired: 7 in, 2 out]
          }
        }
        n72 = Concatenate Strings(w178, w166, w180) -> (w181:string)
        n73 = Bundle By Name(cluster=w170, "OK/NG"=w168) -> (w169:T3)
        n74 = call "FailResumeMode.vi"("NextMessage"="5.2.2_3 Check Environment value from Lux sense", "OK/NG"=w164, "EndMessage"=w163) -> ("OutMessage"=w162:string)  [unwired: 6 in]
        n75 = call "LogStatus.vi"("error in (no error)"=w167, "last message"=w182, "message"=w181) -> ("error  out"=w183:errorcluster)  [unwired: 8 in]
      }
      frame "5.2.2_3 Check Environment value from Lux sense" {
        w212 = FALSE ("x > y?")
        n76 = Unbundle By Name(w223) -> ("Table"=w224:string[][], "OK/NG"=w222:bool)
        n77 = call "Select_Table_Vaule Enable_Disable.vi"("Action"=w225, "Table"=w224) -> ("Enable"=w226:bool)  [unwired: 8 in, 1 out]
        n78 = case shown="假" w226 {
          tunnel: [w233 w244] -> w227
          tunnel: w225 -> [w234 w248]
          tunnel: w224 -> [w235 w247]
          tunnel: w222 -> [w232 w243]
          tunnel: [w232 w242] -> w221
          tunnel: [TRUE ("Result") w241] -> w215
          frame False {
            w239 = "UIdisplay" ("Process (\"\" - local)")
            w233 = "Skip" ("Action")
            n79 = call "Select_Table_Vaule.vi"("Vaule"=w233, "Action"=w234, "Table"=w235) -> ("vaule"=w236:string[])  [unwired: 7 in, 1 out]
            n80 = Build Array (concatenate)(w236, w233, w233) -> (w238:string[])
            n81 = Flatten To XML(anything=w238) -> (xml string=w237:string)
            n82 = call "AMC Send Local Message.vi"("Process (\"\" - local)"=w239, "Message Value"=w237, "Message Name"=w239) -> ()  [unwired: 7 in, 2 out]
          }
          frame True {
            w253 = "UIdisplay" ("Process (\"\" - local)")
            n83 = call "Read_Lux.vi"() -> ("Lux_Value"=w244:string)  [unwired: 9 in, 2 out]
            n84 = call "Select_Table_Vaule.vi"("Vaule"=w244, "Action"=w248, "Table"=w247) -> ("Result"=w241:bool, "vaule"=w246:string[])  [unwired: 7 in]
            n85 = Append True/False String(1:w241, 2:"FAIL" ("真字符串"), 3:"PASS" ("真字符串")) -> (0:w245:string)  [unwired: 1 in]
            n86 = Build Array (concatenate)(w246, w244, w245) -> (w252:string[])
            n87 = And(x=w241, y=w243) -> (x .and. y?=w242:bool)
            n88 = Flatten To XML(anything=w252) -> (xml string=w251:string)
            n89 = call "AMC Send Local Message.vi"("Process (\"\" - local)"=w253, "Message Value"=w251, "Message Name"=w253) -> ()  [unwired: 7 in, 2 out]
          }
        }
        n90 = Concatenate Strings(w225, w218, w227) -> (w228:string)
        n91 = property on="retry_flag" class="Bool (严格)"("Value"=w212) -> ()  [unwired: 2 in, 2 out]
        n92 = property on="GetImage?" class="Bool (严格)"("Value"=w212) -> ()  [unwired: 2 in, 2 out]
        n93 = property on="Num" class="DigNum (严格)"("Value"=0 ("Num")) -> ()  [unwired: 2 in, 2 out]
        n94 = Bundle By Name(cluster=w223, "OK/NG"=w221) -> (w220:T3)
        n95 = call "FailResumeMode.vi"("NextMessage"="SW RESET", "OK/NG"=w215, "EndMessage"=w217) -> ("OutMessage"=w216:string)  [unwired: 6 in]
        n96 = call "LogStatus.vi"("error in (no error)"=w219, "last message"=w229, "message"=w228) -> ("error  out"=w230:errorcluster)  [unwired: 8 in]
      }
      frame "Software Reset" {
        n97 = for {
          N: 3 -> [_]
          tunnel: w264 -> [w295]
          tunnel: [w293] -> w261
          n98 = Unbundle By Name(w295) -> ("NFC _Serial.COM"=w294:refnum<visa-resource-name>)
          n99 = call "NFC_Connect.vi"("VISA resource name"=w294) -> ("NFC"=w293:bool)  [unwired: 9 in, 1 out]
        }
        n100 = case shown="真" w261 {
          tunnel: w272 -> [_ w289]
          tunnel: w270 -> [_ w286]
          tunnel: ["UUT Sleep" w281] -> w269
          frame False {
          }
          frame True {
            n101 = Build Path(base path=w289, name or relative path=w286) -> (appended path=w290:path)
            n102 = call "SendCmd_Tool.vi"("path_bat"=w290) -> ("return code"=w288:i32)  [unwired: 7 in, 7 out]
            n103 = call "NFC_Result.vi"("return code"=w288) -> ("return_result"=w287:string)  [unwired: 9 in, 1 out]
            n104 = call <vilib>:"Trim Whitespace.vi"("string"=w287) -> ("trimmed string"=w285:string)  [unwired: 1 in]
            n105 = Concatenate Strings(w285, "   ", w286) -> (w282:string)
            n106 = flat-sequence {
              tunnel: u32 10000 ("milliseconds to wait") -> [w292]
              tunnel: w282 -> [w291]
              tunnel: [w291] -> w281
              frame #0 {
                n107 = Wait (ms)(milliseconds to wait=w292) -> ()  [unwired: 1 out]
              }
            }
          }
        }
        n108 = call "SW_Config.vi"("Step"=enum16{"Initial", "Write", "Read"}."Read") -> ("SW Config out"=w257:T6)  [unwired: 9 in, 1 out]
        n109 = Unbundle By Name(w257) -> ("682_Tool_Repeat"=w256:string)
        n110 = Decimal String To Number(string=w256) -> (number=w255:i32)  [unwired: 2 in, 1 out]
        n111 = Decrement(x=w255) -> (x-1=w254:i32)
        n112 = property on="Num" class="DigNum (严格)"() -> ("Value"=w268:i32)  [unwired: 2 in, 2 out]
        n113 = Increment(x=w268) -> (x+1=w267:i32)
        n114 = Greater Or Equal?(x=w267, y=w254) -> (x >= y?=→"retry_flag":bool)
        n115 = property on="Num" class="DigNum (严格)"("Value"=w267) -> ()  [unwired: 2 in, 2 out]
        n116 = Concatenate Strings(w275, w273, w269) -> (w276:string)
        n117 = Not(x=w261) -> (.not. x?=w260:bool)
        n118 = call "LogStatus.vi"("error in (no error)"=w274, "last message"=w277, "message"=w276) -> ("error  out"=w278:errorcluster)  [unwired: 8 in]
        n119 = Select(t="5.2.2_4 Start Test mode", s=w261, f=w263) -> (s? t:f=w262:string)
      }
      frame "SW RESET" {
        n120 = for {
          N: 3 -> [_]
          tunnel: w296 -> [w329]
          tunnel: [w327] -> w300
          n121 = Unbundle By Name(w329) -> ("NFC _Serial.COM"=w328:refnum<visa-resource-name>)
          n122 = call "NFC_Connect.vi"("VISA resource name"=w328) -> ("NFC"=w327:bool)  [unwired: 9 in, 1 out]
        }
        n123 = case shown="真" w300 {
          tunnel: w306 -> [_ w323]
          tunnel: w305 -> [_ w320]
          tunnel: ["UUT Sleep" w315] -> w304
          frame False {
          }
          frame True {
            n124 = Build Path(base path=w323, name or relative path=w320) -> (appended path=w324:path)
            n125 = call "SendCmd_Tool.vi"("path_bat"=w324) -> ("return code"=w322:i32)  [unwired: 7 in, 7 out]
            n126 = call "NFC_Result.vi"("return code"=w322) -> ("return_result"=w321:string)  [unwired: 9 in, 1 out]
            n127 = call <vilib>:"Trim Whitespace.vi"("string"=w321) -> ("trimmed string"=w319:string)  [unwired: 1 in]
            n128 = Concatenate Strings(w319, "   ", w320) -> (w316:string)
            n129 = flat-sequence {
              tunnel: u32 10000 ("milliseconds to wait") -> [w326]
              tunnel: w316 -> [w325]
              tunnel: [w325] -> w315
              frame #0 {
                n130 = Wait (ms)(milliseconds to wait=w326) -> ()  [unwired: 1 out]
              }
            }
          }
        }
        n131 = Concatenate Strings(w309, w307, w304) -> (w310:string)
        n132 = Not(x=w300) -> (.not. x?=w299:bool)
        n133 = call "LogStatus.vi"("error in (no error)"=w308, "last message"=w311, "message"=w310) -> ("error  out"=w312:errorcluster)  [unwired: 8 in]
        n134 = Select(t="5.2.2_4 Start Test mode", s=w300, f=w302) -> (s? t:f=w301:string)
      }
      frame "Start Test mode" {
        n135 = Build Path(base path=w339, name or relative path=w336) -> (appended path=w335:path)
        n136 = call "SendCmd_Tool.vi"("path_bat"=w335) -> ("return code"=w334:i32)  [unwired: 7 in, 7 out]
        n137 = call "NFC_Result.vi"("return code"=w334) -> ("return_result"=w333:string)  [unwired: 9 in, 1 out]
        n138 = call <vilib>:"Trim Whitespace.vi"("string"=w333) -> ("trimmed string"=w332:string)  [unwired: 1 in]
        n139 = Concatenate Strings(w332, "   ", w336) -> (w337:string)
        n140 = Concatenate Strings(w342, w340, w337) -> (w343:string)
        n141 = call "LogStatus.vi"("error in (no error)"=w341, "last message"=w344, "message"=w343) -> ("error  out"=w345:errorcluster)  [unwired: 8 in]
      }
      frame "5.2.2_4 Start Test mode" {
        n142 = Unbundle By Name(w356) -> ("Table"=w362:string[][], "OK/NG"=w357:bool)
        n143 = Build Path(base path=w360, name or relative path=w348) -> (appended path=w361:path)
        n144 = call "Select_Table_Vaule Enable_Disable.vi"("Action"=w363, "Table"=w362) -> ("Enable"=w364:bool)  [unwired: 8 in, 1 out]
        n145 = call "SendCmd_Tool.vi"("path_bat"=w361) -> ("return code"=w359:i32, "Other"=w358:string)  [unwired: 7 in, 6 out]
        n146 = case shown="假" w364 {
          tunnel: [w371 w384] -> w365
          tunnel: w363 -> [w371 w397]
          tunnel: w362 -> [w372 w396]
          tunnel: w359 -> [_ w390]
          tunnel: w358 -> [_ w389]
          tunnel: w357 -> [w370 w392]
          tunnel: [w370 w391] -> w354
          tunnel: [TRUE w386] -> w347
          tunnel: w348 -> [_ w383]
          frame False {
            w377 = "UIdisplay" ("Process (\"\" - local)")
            w373 = "Skip" ("Action")
            n147 = call "Select_Table_Vaule.vi"("Vaule"=w373, "Action"=w371, "Table"=w372) -> ("vaule"=w374:string[])  [unwired: 7 in, 1 out]
            n148 = Build Array (concatenate)(w374, w373, w373) -> (w376:string[])
            n149 = Flatten To XML(anything=w376) -> (xml string=w375:string)
            n150 = call "AMC Send Local Message.vi"("Process (\"\" - local)"=w377, "Message Value"=w375, "Message Name"=w377) -> ()  [unwired: 7 in, 2 out]
          }
          frame True {
            n151 = call "NFC_Result.vi"("input"=w389, "return code"=w390) -> ("Command Sucess"=w387:bool, "return_result"=w388:string)  [unwired: 8 in]
            n152 = call <vilib>:"Trim Whitespace.vi"("string"=w388) -> ("trimmed string"=w382:string)  [unwired: 1 in]
            n153 = Concatenate Strings(w383, "   ", w382) -> (w384:string)
            n154 = call "Select_Table_Vaule.vi"("Vaule"=w384, "Action"=w397, "Table"=w396) -> ("Result"=w393:bool, "vaule"=w395:string[])  [unwired: 7 in]
            n155 = And(x=w393, y=w387) -> (x .and. y?=w386:bool)
            n156 = And(x=w386, y=w392) -> (x .and. y?=w391:bool)
            n157 = property on="Num" class="DigNum (严格)"() -> ("Value"=w381:i32)  [unwired: 2 in, 2 out]
            n158 = Append True/False String(1:w386, 2:"FAIL" ("真字符串"), 3:"PASS" ("真字符串")) -> (0:w394:string)  [unwired: 1 in]
            n159 = Less?(x=w381, y=1) -> (x < y?=w379:bool)
            n160 = Build Array (concatenate)(w395, w382, w394) -> (w401:string[])
            n161 = Flatten To XML(anything=w401) -> (xml string=w400:string)
            n162 = case shown="真" w379 {
              tunnel: w400 -> [_ w402]
              frame False {
              }
              frame True {
                w403 = "UIdisplay" ("Process (\"\" - local)")
                n163 = call "AMC Send Local Message.vi"("Process (\"\" - local)"=w403, "Message Value"=w402, "Message Name"=w403) -> ()  [unwired: 7 in, 2 out]
              }
            }
          }
        }
        n164 = Concatenate Strings(w363, w352, w365) -> (w366:string)
        n165 = call "FailResumeMode.vi"("NextMessage"="5.2.2_5 Start camera test mode", "OK/NG"=w347, "EndMessage"=w350) -> ("OutMessage"=w349:string)  [unwired: 6 in]
        n166 = Bundle By Name(cluster=w356, "OK/NG"=w354) -> (w355:T3)
        n167 = call "LogStatus.vi"("error in (no error)"=w353, "last message"=w367, "message"=w366) -> ("error  out"=w368:errorcluster)  [unwired: 8 in]
      }
      frame "5.2.2_5 Start camera test mode" {
        n168 = Unbundle By Name(w415) -> ("Table"=w419:string[][], "OK/NG"=w416:bool)
        n169 = Build Path(base path=w417, name or relative path=w404) -> (appended path=w418:path)
        n170 = call "SendCmd_Tool.vi"("path_bat"=w418) -> ("return code"=w412:i32, "Other"=w411:string)  [unwired: 7 in, 6 out]
        n171 = call "Select_Table_Vaule Enable_Disable.vi"("Action"=w420, "Table"=w419) -> ("Enable"=w421:bool)  [unwired: 8 in, 1 out]
        n172 = case shown="假" w421 {
          tunnel: [w428 w442] -> w422
          tunnel: w420 -> [w429 w454]
          tunnel: w419 -> [w430 w453]
          tunnel: w412 -> [_ w447]
          tunnel: w416 -> [w427 w449]
          tunnel: [w427 w448] -> w413
          tunnel: w411 -> [_ w446]
          tunnel: [TRUE w444] -> w408
          tunnel: w404 -> [_ w436]
          frame False {
            w434 = "UIdisplay" ("Process (\"\" - local)")
            w428 = "Skip" ("Action")
            n173 = call "Select_Table_Vaule.vi"("Vaule"=w428, "Action"=w429, "Table"=w430) -> ("vaule"=w431:string[])  [unwired: 7 in, 1 out]
            n174 = Build Array (concatenate)(w431, w428, w428) -> (w433:string[])
            n175 = Flatten To XML(anything=w433) -> (xml string=w432:string)
            n176 = call "AMC Send Local Message.vi"("Process (\"\" - local)"=w434, "Message Value"=w432, "Message Name"=w434) -> ()  [unwired: 7 in, 2 out]
          }
          frame True {
            n177 = call "NFC_Result.vi"("input"=w446, "return code"=w447) -> ("Command Sucess"=w440:bool, "return_result"=w445:string)  [unwired: 8 in]
            n178 = call <vilib>:"Trim Whitespace.vi"("string"=w445) -> ("trimmed string"=w441:string)  [unwired: 1 in]
            n179 = Concatenate Strings(w436, "   ", w441) -> (w442:string)
            n180 = call "Select_Table_Vaule.vi"("Vaule"=w442, "Action"=w454, "Table"=w453) -> ("Result"=w450:bool, "vaule"=w452:string[])  [unwired: 7 in]
            n181 = And(x=w450, y=w440) -> (x .and. y?=w444:bool)
            n182 = Append True/False String(1:w444, 2:"FAIL" ("真字符串"), 3:"PASS" ("真字符串")) -> (0:w451:string)  [unwired: 1 in]
            n183 = property on="Num" class="DigNum (严格)"() -> ("Value"=w439:i32)  [unwired: 2 in, 2 out]
            n184 = Less?(x=w439, y=1) -> (x < y?=w437:bool)
            n185 = Build Array (concatenate)(w452, w441, w451) -> (w458:string[])
            n186 = Flatten To XML(anything=w458) -> (xml string=w457:string)
            n187 = case shown="真" w437 {
              tunnel: w457 -> [_ w460]
              frame False {
              }
              frame True {
                w459 = "UIdisplay" ("Process (\"\" - local)")
                n188 = call "AMC Send Local Message.vi"("Process (\"\" - local)"=w459, "Message Value"=w460, "Message Name"=w459) -> ()  [unwired: 7 in, 2 out]
              }
            }
            n189 = And(x=w444, y=w449) -> (x .and. y?=w448:bool)
          }
        }
        n190 = Concatenate Strings(w420, w409, w422) -> (w423:string)
        n191 = Bundle By Name(cluster=w415, "OK/NG"=w413) -> (w414:T3)
        n192 = call "FailResumeMode.vi"("NextMessage"="5.2.2_6 get one RAW Image", "OK/NG"=w408, "EndMessage"=w406) -> ("OutMessage"=w405:string)  [unwired: 6 in]
        n193 = call "LogStatus.vi"("error in (no error)"=w410, "last message"=w424, "message"=w423) -> ("error  out"=w425:errorcluster)  [unwired: 8 in]
      }
      frame "5.2.2_6 get one RAW Image" {
        (unwired) "5.2.2_9 Write back calibration data to UUT"
        n194 = Unbundle By Name(w478) -> ("Table"=w482:string[][], "OK/NG"=w479:bool, "SN"=w464:string)
        n195 = Build Path(base path=w472, name or relative path=w461) -> (appended path=w465:path)
        n196 = call "Calibration_Image_Save.vi"("SN"=w464, "file"=w465) -> ("error out"=w463:errorcluster, "path"=w462:path)  [unwired: 8 in]
        n197 = call "SendCmd_Tool.vi"("path_bat"=w462, "error in (no error) 2"=w463) -> ("VQT"=w466:string, "return code"=w481:i32, "Other"=w480:string)  [unwired: 6 in, 5 out]
        n198 = call "Select_Table_Vaule Enable_Disable.vi"("Action"=w483, "Table"=w482) -> ("Enable"=w484:bool)  [unwired: 8 in, 1 out]
        n199 = case shown="假" w484 {
          tunnel: [w491 w505] -> w485
          tunnel: w483 -> [w492 w517]
          tunnel: w482 -> [w493 w516]
          tunnel: w481 -> [_ w511]
          tunnel: w480 -> [_ w510]
          tunnel: w479 -> [w490 w506]
          tunnel: [w490 w512] -> w471
          tunnel: [TRUE w500] -> w468
          tunnel: w461 -> [_ w507]
          tunnel: w466 -> [_ w501]
          frame False {
            w497 = "UIdisplay" ("Process (\"\" - local)")
            w491 = "Skip" ("Action")
            n200 = call "Select_Table_Vaule.vi"("Vaule"=w491, "Action"=w492, "Table"=w493) -> ("vaule"=w494:string[])  [unwired: 7 in, 1 out]
            n201 = Build Array (concatenate)(w494, w491, w491) -> (w496:string[])
            n202 = Flatten To XML(anything=w496) -> (xml string=w495:string)
            n203 = call "AMC Send Local Message.vi"("Process (\"\" - local)"=w497, "Message Value"=w495, "Message Name"=w497) -> ()  [unwired: 7 in, 2 out]
          }
          frame True {
            w502 = "   "
            n204 = call "NFC_Result.vi"("input"=w510, "return code"=w511) -> ("Command Sucess"=w499:bool, "return_result"=w509:string)  [unwired: 8 in]
            "GetImage?" <- w499
            n205 = call <vilib>:"Trim Whitespace.vi"("string"=w509) -> ("trimmed string"=w504:string)  [unwired: 1 in]
            n206 = Concatenate Strings(w507, w502, w504, w502, w501) -> (w505:string)
            n207 = call "Select_Table_Vaule.vi"("Vaule"=w505, "Action"=w517, "Table"=w516) -> ("Result"=w513:bool, "vaule"=w515:string[])  [unwired: 7 in]
            n208 = And(x=w513, y=w499) -> (x .and. y?=w508:bool)
            n209 = property on="retry_flag" class="Bool (严格)"() -> ("Value"=w503:bool)  [unwired: 2 in, 2 out]
            n210 = Append True/False String(1:w508, 2:"FAIL" ("真字符串"), 3:"PASS" ("真字符串")) -> (0:w514:string)  [unwired: 1 in]
            n211 = Or(x=w499, y=w503) -> (x .or. y?=w500:bool)
            n212 = case shown="真" w500 {
              tunnel: w515 -> [_ w522]
              tunnel: w514 -> [_ w521]
              tunnel: w504 -> [_ w520]
              frame False {
              }
              frame True {
                w525 = "UIdisplay" ("Process (\"\" - local)")
                n213 = Build Array (concatenate)(w522, w520, w521) -> (w524:string[])
                n214 = Flatten To XML(anything=w524) -> (xml string=w523:string)
                n215 = call "AMC Send Local Message.vi"("Process (\"\" - local)"=w525, "Message Value"=w523, "Message Name"=w525) -> ()  [unwired: 7 in, 2 out]
              }
            }
            n216 = And(x=w508, y=w506) -> (x .and. y?=w512:bool)
          }
        }
        n217 = Concatenate Strings(w483, w475, w485) -> (w486:string)
        n218 = Bundle By Name(cluster=w478, "OK/NG"=w471) -> (w477:T3)
        n219 = Select(t="5.2.2_7 Find Image  in the CLI tool directory", s=w468, f="Software Reset") -> (s? t:f=w469:string)
        n220 = call "LogStatus.vi"("error in (no error)"=w476, "last message"=w487, "message"=w486) -> ("error  out"=w488:errorcluster)  [unwired: 8 in]
        n221 = call "FailResumeMode.vi"("NextMessage"=w469, "OK/NG"=w468, "EndMessage"=w474) -> ("OutMessage"=w473:string)  [unwired: 6 in]
      }
      frame "5.2.2_7 Find Image  in the CLI tool directory" {
        n222 = Unbundle By Name(w532) -> ("Table"=w536:string[][], "OK/NG"=w529:bool)
        n223 = call "Select_Table_Vaule Enable_Disable.vi"("Action"=w537, "Table"=w536) -> ("Enable"=w538:bool)  [unwired: 8 in, 1 out]
        n224 = case shown="真" w538 {
          tunnel: [w546 w557] -> w539
          tunnel: w537 -> [w547 w562]
          tunnel: w536 -> [w548 w561]
          tunnel: [TRUE ("Result") w555] -> w531
          tunnel: w529 -> [w545 w554]
          tunnel: [w545 w553] -> w528
          frame False {
            w552 = "UIdisplay" ("Process (\"\" - local)")
            w546 = "Skip" ("Action")
            n225 = call "Select_Table_Vaule.vi"("Vaule"=w546, "Action"=w547, "Table"=w548) -> ("vaule"=w549:string[])  [unwired: 7 in, 1 out]
            n226 = Build Array (concatenate)(w549, w546, w546) -> (w551:string[])
            n227 = Flatten To XML(anything=w551) -> (xml string=w550:string)
            n228 = call "AMC Send Local Message.vi"("Process (\"\" - local)"=w552, "Message Value"=w550, "Message Name"=w552) -> ()  [unwired: 7 in, 2 out]
          }
          frame True {
            w567 = "UIdisplay" ("Process (\"\" - local)")
            n229 = property on="GetImage?" class="Bool (严格)"() -> ("Value"=w555:bool)  [unwired: 2 in, 2 out]
            n230 = Select(t="Yes" ("response"), s=w555, f="No" ("response")) -> (s? t:f=w557:string)
            n231 = call "Select_Table_Vaule.vi"("Vaule"=w557, "Action"=w562, "Table"=w561) -> ("vaule"=w560:string[])  [unwired: 7 in, 1 out]
            n232 = Append True/False String(1:w555, 2:"FAIL" ("真字符串"), 3:"PASS" ("真字符串")) -> (0:w556:string)  [unwired: 1 in]
            n233 = And(x=w555, y=w554) -> (x .and. y?=w553:bool)
            n234 = Build Array (concatenate)(w560, w557, w556) -> (w566:string[])
            n235 = Flatten To XML(anything=w566) -> (xml string=w565:string)
            n236 = call "AMC Send Local Message.vi"("Process (\"\" - local)"=w567, "Message Value"=w565, "Message Name"=w567) -> ()  [unwired: 7 in, 2 out]
          }
        }
        n237 = Concatenate Strings(w537, w534, w539) -> (w540:string)
        n238 = Bundle By Name(cluster=w532, "OK/NG"=w528) -> (w530:T3)
        n239 = call "FailResumeMode.vi"("NextMessage"="5.2.2_9 Write black calibration data to UUT", "OK/NG"=w531, "EndMessage"=w533) -> ("OutMessage"=w526:string)  [unwired: 6 in]
        n240 = call "LogStatus.vi"("error in (no error)"=w535, "last message"=w541, "message"=w540) -> ("error  out"=w542:errorcluster)  [unwired: 8 in]
      }
      frame "5.2.2_9 Write black calibration data to UUT" {
        n241 = Unbundle By Name(w575) -> ("Table"=w583:string[][], "OK/NG"=w576:bool)
        n242 = Build Path(base path=w578, name or relative path=w570) -> (appended path=w579:path)
        n243 = call "SendCmd_Tool.vi"("path_bat"=w579) -> ("return code"=w577:i32, "Other"=w572:string)  [unwired: 7 in, 6 out]
        n244 = call "Select_Table_Vaule Enable_Disable.vi"("Action"=w584, "Table"=w583) -> ("Enable"=w585:bool)  [unwired: 8 in, 1 out]
        n245 = case shown="假" w585 {
          tunnel: [w592 w603] -> w586
          tunnel: w584 -> [w593 w616]
          tunnel: w583 -> [w594 w615]
          tunnel: [TRUE ("Result") w608] -> w580
          tunnel: w577 -> [_ w602]
          tunnel: w576 -> [w591 w611]
          tunnel: [w591 w607] -> w573
          tunnel: w572 -> [_ w606]
          tunnel: w570 -> [_ w600]
          frame False {
            w598 = "UIdisplay" ("Process (\"\" - local)")
            w592 = "Skip" ("Action")
            n246 = call "Select_Table_Vaule.vi"("Vaule"=w592, "Action"=w593, "Table"=w594) -> ("vaule"=w595:string[])  [unwired: 7 in, 1 out]
            n247 = Build Array (concatenate)(w595, w592, w592) -> (w597:string[])
            n248 = Flatten To XML(anything=w597) -> (xml string=w596:string)
            n249 = call "AMC Send Local Message.vi"("Process (\"\" - local)"=w598, "Message Value"=w596, "Message Name"=w598) -> ()  [unwired: 7 in, 2 out]
          }
          frame True {
            w621 = "UIdisplay" ("Process (\"\" - local)")
            n250 = call "NFC_Result.vi"("input"=w606, "return code"=w602) -> ("Command Sucess"=w610:bool, "return_result"=w612:string)  [unwired: 8 in]
            n251 = call <vilib>:"Trim Whitespace.vi"("string"=w612) -> ("trimmed string"=w604:string)  [unwired: 1 in]
            n252 = Concatenate Strings(w600, "   ", w604) -> (w603:string)
            n253 = Number To Decimal String(number=w602) -> (decimal integer string=w601:string)  [unwired: 1 in]
            n254 = call "Select_Table_Vaule.vi"("Vaule"=w603, "Action"=w616, "Table"=w615) -> ("Result"=w609:bool, "vaule"=w614:string[])  [unwired: 7 in]
            n255 = And(x=w609, y=w610) -> (x .and. y?=w608:bool)
            n256 = Append True/False String(1:w608, 2:"FAIL" ("真字符串"), 3:"PASS" ("真字符串")) -> (0:w613:string)  [unwired: 1 in]
            n257 = And(x=w608, y=w611) -> (x .and. y?=w607:bool)
            n258 = Build Array (concatenate)(w614, w601, w613) -> (w620:string[])
            n259 = Flatten To XML(anything=w620) -> (xml string=w619:string)
            n260 = call "AMC Send Local Message.vi"("Process (\"\" - local)"=w621, "Message Value"=w619, "Message Name"=w621) -> ()  [unwired: 7 in, 2 out]
          }
        }
        n261 = Concatenate Strings(w584, w581, w586) -> (w587:string)
        n262 = call "FailResumeMode.vi"("NextMessage"="5.2.2_10 Stop camera test mode", "OK/NG"=w580, "EndMessage"=w571) -> ("OutMessage"=w568:string)  [unwired: 6 in]
        n263 = Bundle By Name(cluster=w575, "OK/NG"=w573) -> (w574:T3)
        n264 = call "LogStatus.vi"("error in (no error)"=w582, "last message"=w588, "message"=w587) -> ("error  out"=w589:errorcluster)  [unwired: 8 in]
      }
      frame "5.2.2_10 Stop camera test mode" {
        n265 = Unbundle By Name(w630) -> ("Table"=w637:string[][], "OK/NG"=w631:bool)
        n266 = Build Path(base path=w635, name or relative path=w634) -> (appended path=w636:path)
        n267 = call "SendCmd_Tool.vi"("path_bat"=w636) -> ("return code"=w633:i32, "Other"=w632:string)  [unwired: 7 in, 6 out]
        n268 = call "Select_Table_Vaule Enable_Disable.vi"("Action"=w638, "Table"=w637) -> ("Enable"=w639:bool)  [unwired: 8 in, 1 out]
        n269 = case shown="假" w639 {
          tunnel: [w646 w654] -> w640
          tunnel: w638 -> [w646 w666]
          tunnel: w637 -> [w647 w665]
          tunnel: w633 -> [_ w658]
          tunnel: w632 -> [_ w657]
          tunnel: w631 -> [w645 w661]
          tunnel: [w645 w660] -> w628
          tunnel: [TRUE w655] -> w623
          frame False {
            w652 = "UIdisplay" ("Process (\"\" - local)")
            w648 = "Skip" ("Action")
            n270 = call "Select_Table_Vaule.vi"("Vaule"=w648, "Action"=w646, "Table"=w647) -> ("vaule"=w649:string[])  [unwired: 7 in, 1 out]
            n271 = Build Array (concatenate)(w649, w648, w648) -> (w651:string[])
            n272 = Flatten To XML(anything=w651) -> (xml string=w650:string)
            n273 = call "AMC Send Local Message.vi"("Process (\"\" - local)"=w652, "Message Value"=w650, "Message Name"=w652) -> ()  [unwired: 7 in, 2 out]
          }
          frame True {
            w671 = "UIdisplay" ("Process (\"\" - local)")
            n274 = call "NFC_Result.vi"("input"=w657, "return code"=w658) -> ("Command Sucess"=w656:bool, "return_result"=w659:string)  [unwired: 8 in]
            n275 = call <vilib>:"Trim Whitespace.vi"("string"=w659) -> ("trimmed string"=w654:string)  [unwired: 1 in]
            n276 = call "Select_Table_Vaule.vi"("Vaule"=w654, "Action"=w666, "Table"=w665) -> ("Result"=w662:bool, "vaule"=w664:string[])  [unwired: 7 in]
            n277 = And(x=w662, y=w656) -> (x .and. y?=w655:bool)
            n278 = And(x=w655, y=w661) -> (x .and. y?=w660:bool)
            n279 = Append True/False String(1:w655, 2:"FAIL" ("真字符串"), 3:"PASS" ("真字符串")) -> (0:w663:string)  [unwired: 1 in]
            n280 = Build Array (concatenate)(w664, w654, w663) -> (w670:string[])
            n281 = Flatten To XML(anything=w670) -> (xml string=w669:string)
            n282 = call "AMC Send Local Message.vi"("Process (\"\" - local)"=w671, "Message Value"=w669, "Message Name"=w671) -> ()  [unwired: 7 in, 2 out]
          }
        }
        n283 = Concatenate Strings(w638, w626, w640) -> (w641:string)
        n284 = Bundle By Name(cluster=w630, "OK/NG"=w628) -> (w629:T3)
        n285 = call "FailResumeMode.vi"("NextMessage"="5.2.2_11 Stop Test Mode", "OK/NG"=w623, "EndMessage"=w624) -> ("OutMessage"=w622:string)  [unwired: 6 in]
        n286 = call "LogStatus.vi"("error in (no error)"=w627, "last message"=w642, "message"=w641) -> ("error  out"=w643:errorcluster)  [unwired: 8 in]
      }
      frame "5.2.2_11 Stop Test Mode" {
        n287 = Unbundle By Name(w680) -> ("Table"=w687:string[][], "OK/NG"=w681:bool)
        n288 = Build Path(base path=w685, name or relative path=w684) -> (appended path=w686:path)
        n289 = call "SendCmd_Tool.vi"("path_bat"=w686) -> ("return code"=w682:i32, "Other"=w683:string)  [unwired: 7 in, 6 out]
        n290 = call "Select_Table_Vaule Enable_Disable.vi"("Action"=w688, "Table"=w687) -> ("Enable"=w689:bool)  [unwired: 8 in, 1 out]
        n291 = case shown="假" w689 {
          tunnel: [w696 w709] -> w690
          tunnel: w688 -> [w696 w716]
          tunnel: w687 -> [w697 w715]
          tunnel: w683 -> [_ w707]
          tunnel: w682 -> [_ w708]
          tunnel: w681 -> [w695 w711]
          tunnel: [w695 w710] -> w678
          tunnel: [TRUE w704] -> w674
          frame False {
            w702 = "UIdisplay" ("Process (\"\" - local)")
            w698 = "Skip" ("Action")
            n292 = call "Select_Table_Vaule.vi"("Vaule"=w698, "Action"=w696, "Table"=w697) -> ("vaule"=w699:string[])  [unwired: 7 in, 1 out]
            n293 = Build Array (concatenate)(w699, w698, w698) -> (w701:string[])
            n294 = Flatten To XML(anything=w701) -> (xml string=w700:string)
            n295 = call "AMC Send Local Message.vi"("Process (\"\" - local)"=w702, "Message Value"=w700, "Message Name"=w702) -> ()  [unwired: 7 in, 2 out]
          }
          frame True {
            w721 = "UIdisplay" ("Process (\"\" - local)")
            n296 = call "NFC_Result.vi"("input"=w707, "return code"=w708) -> ("Command Sucess"=w706:bool, "return_result"=w705:string)  [unwired: 8 in]
            n297 = call <vilib>:"Trim Whitespace.vi"("string"=w705) -> ("trimmed string"=w709:string)  [unwired: 1 in]
            n298 = call "Select_Table_Vaule.vi"("Vaule"=w709, "Action"=w716, "Table"=w715) -> ("Result"=w712:bool, "vaule"=w714:string[])  [unwired: 7 in]
            n299 = And(x=w712, y=w706) -> (x .and. y?=w704:bool)
            n300 = Append True/False String(1:w704, 2:"FAIL" ("真字符串"), 3:"PASS" ("真字符串")) -> (0:w713:string)  [unwired: 1 in]
            n301 = And(x=w704, y=w711) -> (x .and. y?=w710:bool)
            n302 = Build Array (concatenate)(w714, w709, w713) -> (w720:string[])
            n303 = Flatten To XML(anything=w720) -> (xml string=w719:string)
            n304 = call "AMC Send Local Message.vi"("Process (\"\" - local)"=w721, "Message Value"=w719, "Message Name"=w721) -> ()  [unwired: 7 in, 2 out]
          }
        }
        n305 = Concatenate Strings(w688, w676, w690) -> (w691:string)
        n306 = Bundle By Name(cluster=w680, "OK/NG"=w678) -> (w679:T3)
        n307 = call "FailResumeMode.vi"("NextMessage"="5.2.2_12 Reboot UUT by EOL Test Command", "OK/NG"=w674, "EndMessage"=w673) -> ("OutMessage"=w672:string)  [unwired: 6 in]
        n308 = call "LogStatus.vi"("error in (no error)"=w677, "last message"=w692, "message"=w691) -> ("error  out"=w693:errorcluster)  [unwired: 8 in]
      }
      frame "5.2.2_12 Reboot UUT by EOL Test Command" {
        # "Pass"
        n309 = Unbundle By Name(w728) -> ("Table"=w737:string[][], "OK/NG"=w726:bool)
        n310 = call "Select_Table_Vaule Enable_Disable.vi"("Action"=w738, "Table"=w737) -> ("Enable"=w725:bool)  [unwired: 8 in, 1 out]
        n311 = case shown="假" w725 {
          tunnel: [w745 w759] -> w739
          tunnel: w738 -> [w746 w773]
          tunnel: w737 -> [w747 w772]
          tunnel: [w744 w753] -> w729
          tunnel: w733 -> [_ _]
          tunnel: w731 -> [_ w761]
          tunnel: w730 -> [_ w760]
          tunnel: w726 -> [w744 w754]
          tunnel: [TRUE w752] -> w722
          frame False {
            w751 = "UIdisplay" ("Process (\"\" - local)")
            w745 = "Skip" ("Action")
            n312 = call "Select_Table_Vaule.vi"("Vaule"=w745, "Action"=w746, "Table"=w747) -> ("vaule"=w748:string[])  [unwired: 7 in, 1 out]
            n313 = Build Array (concatenate)(w748, w745, w745) -> (w750:string[])
            n314 = Flatten To XML(anything=w750) -> (xml string=w749:string)
            n315 = call "AMC Send Local Message.vi"("Process (\"\" - local)"=w751, "Message Value"=w749, "Message Name"=w751) -> ()  [unwired: 7 in, 2 out]
          }
          frame True {
            w778 = "UIdisplay" ("Process (\"\" - local)")
            n316 = Build Path(base path=w761, name or relative path=w760) -> (appended path=w768:path)
            n317 = call "SendCmd_Tool.vi"("path_bat"=w768) -> ("return code"=w767:i32)  [unwired: 7 in, 7 out]
            n318 = call "NFC_Result.vi"("return code"=w767) -> ("Command Sucess"=w756:bool, "return_result"=w766:string)  [unwired: 9 in]
            n319 = call <vilib>:"Trim Whitespace.vi"("string"=w766) -> ("trimmed string"=w765:string)  [unwired: 1 in]
            n320 = Concatenate Strings(w765, "   ", w760) -> (w762:string)
            n321 = flat-sequence {
              tunnel: u32 10000 ("milliseconds to wait") -> [w780]
              tunnel: w762 -> [w779]
              tunnel: [w779] -> w759
              frame #0 {
                n322 = Wait (ms)(milliseconds to wait=w780) -> ()  [unwired: 1 out]
              }
            }
            n323 = Select(t="Pass" ("response"), s=w756, f="Fail" ("response")) -> (s? t:f=w755:string)
            n324 = call "Select_Table_Vaule.vi"("Vaule"=w759, "Action"=w773, "Table"=w772) -> ("Result"=w770:bool, "vaule"=w771:string[])  [unwired: 7 in]
            n325 = And(x=w770, y=w756) -> (x .and. y?=w752:bool)
            n326 = Append True/False String(1:w752, 2:"FAIL" ("真字符串"), 3:"PASS" ("真字符串")) -> (0:w769:string)  [unwired: 1 in]
            n327 = Build Array (concatenate)(w771, w755, w769) -> (w777:string[])
            n328 = And(x=w752, y=w754) -> (x .and. y?=w753:bool)
            n329 = Flatten To XML(anything=w777) -> (xml string=w776:string)
            n330 = call "AMC Send Local Message.vi"("Process (\"\" - local)"=w778, "Message Value"=w776, "Message Name"=w778) -> ()  [unwired: 7 in, 2 out]
          }
        }
        n331 = Concatenate Strings(w738, w735, w739) -> (w732:string)
        n332 = Bundle By Name(cluster=w728, "OK/NG"=w729) -> (w727:T3)
        n333 = call "LogStatus.vi"("error in (no error)"=w736, "last message"=w740, "message"=w732) -> ("error  out"=w741:errorcluster)  [unwired: 8 in]
        n334 = call "FailResumeMode.vi"("NextMessage"="Start Test mode", "OK/NG"=w722, "EndMessage"=w734) -> ("OutMessage"=w723:string)  [unwired: 6 in]
      }
      frame "5.2.2_13 Re-connect UUT by NFC" {
        n335 = Unbundle By Name(w787) -> ("Table"=w793:string[][], "OK/NG"=w784:bool)
        n336 = call "Select_Table_Vaule Enable_Disable.vi"("Action"=w794, "Table"=w793) -> ("Enable"=w782:bool)  [unwired: 8 in, 1 out]
        n337 = case shown="真" w782 {
          tunnel: [w801 w812] -> w795
          tunnel: w794 -> [w801 w823]
          tunnel: w793 -> [w802 w822]
          tunnel: [TRUE ("Result") w811] -> w786
          tunnel: w788 -> [_ w815]
          tunnel: w784 -> [w800 w810]
          tunnel: [w800 w809] -> w783
          frame False {
            w807 = "UIdisplay" ("Process (\"\" - local)")
            w803 = "Skip" ("Action")
            n338 = call "Select_Table_Vaule.vi"("Vaule"=w803, "Action"=w801, "Table"=w802) -> ("vaule"=w804:string[])  [unwired: 7 in, 1 out]
            n339 = Build Array (concatenate)(w804, w803, w803) -> (w806:string[])
            n340 = Flatten To XML(anything=w806) -> (xml string=w805:string)
            n341 = call "AMC Send Local Message.vi"("Process (\"\" - local)"=w807, "Message Value"=w805, "Message Name"=w807) -> ()  [unwired: 7 in, 2 out]
          }
          frame True {
            w827 = "UIdisplay" ("Process (\"\" - local)")
            n342 = for {
              N: 3 -> [_]
              tunnel: w815 -> [w830]
              tunnel: [w828] -> w818
              n343 = Unbundle By Name(w830) -> ("NFC _Serial.COM"=w829:refnum<visa-resource-name>)
              n344 = call "NFC_Connect.vi"("VISA resource name"=w829) -> ("NFC"=w828:bool)  [unwired: 9 in, 1 out]
            }
            n345 = Select(t="Pass" ("response"), s=w818, f="Fail" ("response")) -> (s? t:f=w812:string)
            n346 = call "Select_Table_Vaule.vi"("Vaule"=w812, "Action"=w823, "Table"=w822) -> ("Result"=w813:bool, "vaule"=w821:string[])  [unwired: 7 in]
            n347 = And(x=w813, y=w818) -> (x .and. y?=w811:bool)
            n348 = And(x=w811, y=w810) -> (x .and. y?=w809:bool)
            n349 = Append True/False String(1:w811, 2:"FAIL" ("真字符串"), 3:"PASS" ("真字符串")) -> (0:w814:string)  [unwired: 1 in]
            n350 = Build Array (concatenate)(w821, w812, w814) -> (w826:string[])
            n351 = Flatten To XML(anything=w826) -> (xml string=w825:string)
            n352 = call "AMC Send Local Message.vi"("Process (\"\" - local)"=w827, "Message Value"=w825, "Message Name"=w827) -> ()  [unwired: 7 in, 2 out]
          }
        }
        n353 = Concatenate Strings(w794, w791, w795) -> (w796:string)
        n354 = Bundle By Name(cluster=w787, "OK/NG"=w783) -> (w785:T3)
        n355 = call "FailResumeMode.vi"("NextMessage"="5.2.2_14 verify OBC setting by EOL Test command", "OK/NG"=w786, "EndMessage"=w790) -> ("OutMessage"=w781:string)  [unwired: 6 in]
        n356 = call "LogStatus.vi"("error in (no error)"=w792, "last message"=w797, "message"=w796) -> ("error  out"=w798:errorcluster)  [unwired: 8 in]
      }
      frame "5.2.2_14 verify OBC setting by EOL Test command" {
        n357 = Unbundle By Name(w836) -> ("Table"=w845:string[][], "OK/NG"=w833:bool)
        n358 = call "Select_Table_Vaule Enable_Disable.vi"("Action"=w846, "Table"=w845) -> ("Enable"=w831:bool)  [unwired: 8 in, 1 out]
        n359 = case shown="真" w831 {
          tunnel: [w855 w870] -> w847
          tunnel: w846 -> [w853 w878]
          tunnel: w845 -> [w854 w877]
          tunnel: [TRUE ("Result") w865] -> w835
          tunnel: w838 -> [_ w872]
          tunnel: w837 -> [_ w871]
          tunnel: w833 -> [w852 w864]
          tunnel: [w852 w863] -> w832
          frame False {
            w859 = "UIdisplay" ("Process (\"\" - local)")
            w855 = "Skip" ("Action")
            n360 = call "Select_Table_Vaule.vi"("Vaule"=w855, "Action"=w853, "Table"=w854) -> ("vaule"=w856:string[])  [unwired: 7 in, 1 out]
            n361 = Build Array (concatenate)(w856, w855, w855) -> (w858:string[])
            n362 = Flatten To XML(anything=w858) -> (xml string=w857:string)
            n363 = call "AMC Send Local Message.vi"("Process (\"\" - local)"=w859, "Message Value"=w857, "Message Name"=w859) -> ()  [unwired: 7 in, 2 out]
          }
          frame True {
            w883 = "UIdisplay" ("Process (\"\" - local)")
            n364 = Build Path(base path=w872, name or relative path=w871) -> (appended path=w875:path)
            n365 = call "SendCmd_Tool.vi"("path_bat"=w875) -> ("return code"=w874:i32, "Other"=w861:string)  [unwired: 7 in, 6 out]
            n366 = call "NFC_Result.vi"("input"=w861, "return code"=w874) -> ("Command Sucess"=w866:bool, "return_result"=w862:string)  [unwired: 8 in]
            n367 = call <vilib>:"Trim Whitespace.vi"("string"=w862) -> ("trimmed string"=w868:string)  [unwired: 1 in]
            n368 = Concatenate Strings(w868, "   ", w871) -> (w870:string)
            n369 = call "Select_Table_Vaule.vi"("Vaule"=w870, "Action"=w878, "Table"=w877) -> ("Result"=w867:bool, "vaule"=w876:string[])  [unwired: 7 in]
            n370 = And(x=w867, y=w866) -> (x .and. y?=w865:bool)
            n371 = Append True/False String(1:w865, 2:"FAIL" ("真字符串"), 3:"PASS" ("真字符串")) -> (0:w869:string)  [unwired: 1 in]
            n372 = Build Array (concatenate)(w876, w868, w869) -> (w882:string[])
            n373 = And(x=w865, y=w864) -> (x .and. y?=w863:bool)
            n374 = Flatten To XML(anything=w882) -> (xml string=w881:string)
            n375 = call "AMC Send Local Message.vi"("Process (\"\" - local)"=w883, "Message Value"=w881, "Message Name"=w883) -> ()  [unwired: 7 in, 2 out]
          }
        }
        n376 = Concatenate Strings(w846, w842, w847) -> (w848:string)
        n377 = call "FailResumeMode.vi"("NextMessage"="5.2.3_Camera Vision Quality Test", "OK/NG"=w835, "EndMessage"=w839) -> ("OutMessage"=w840:string)  [unwired: 6 in]
        n378 = Bundle By Name(cluster=w836, "OK/NG"=w832) -> (w834:T3)
        n379 = call "LogStatus.vi"("error in (no error)"=w843, "last message"=w849, "message"=w848) -> ("error  out"=w850:errorcluster)  [unwired: 8 in]
      }
    }
    n380 = call "Stop.vi"("Step"=enum16{"Initial", "Write", "Read"}."Read") -> ("Stop Out"=w52:bool)  [unwired: 9 in, 1 out]
    n381 = call "Exit.vi"("Step"=enum16{"Initial", "Write", "Read"}."Read" ("step")) -> ("Exit Out"=w51:bool)  [unwired: 9 in, 1 out]
    n382 = call "6-AlarmStatus.vi"("Step"=enum16{"Initial", "Write", "Read"}."Read") -> ("AlarmValue Out"=w44:bool[])  [unwired: 9 in, 1 out]
    n383 = Or Array Elements(Boolean array=w44) -> (logical OR=w43:bool)
    n384 = Compound Arithmetic op=OR(w50, w52, w51, w43) -> (w49:bool)
    n385 = call "AMC Run Step.vi"("Message Queue In"=w67, "Message Name"=w57, "Message Value"=w55, "error in (no error)"=w62, "Mli/Sig"=FALSE) -> ("Message Queue Out"=w66:T4, "error out"=w61:errorcluster)  [unwired: 13 in]
  }
  "Message Queue Out" <- w23
  "error out" <- w22
  "Data out" <- w20
